vi "Autonomous Independent.vi"() -> ()   [LabVIEW 2012]
doc: "This VI is called when autonomous begins, and will automatically be terminated when autonomous ends. You can carry out timed or sensor driven robot movement independently without needing to return to the caller."
uses:
  <vilib>/Rock Robotics/WPI/Relay/WPI_RelayValue.ctl
  <vilib>/Rock Robotics/WPI/RobotDrive/WPI_RobotDriveGetSetRefNum.vi
  Robot Global Data.vi
panel:
  out "Shooter Up":bool
  out "Shooter Speed":T1(ring)
  out "Stop Drive":bool
  out "DT Output":enum16{"Off", "Up", "Down"}(ring)=enum."Down"
  out "DAD Up":bool
  out "DAD Output":T2
  out "Shift Low":bool
  out "Feeder Happy":bool
  out "Auton Done":bool
  out "Shooter Happy":bool
  out "Shoot!":bool
  out "Delay Switch":u32
  out "Seccond Switch":u32
  out "First Switch":u32
  # "Be sure to right-click and choose Data Operations>>Make Current Value default if you want to save the array values with the VI"
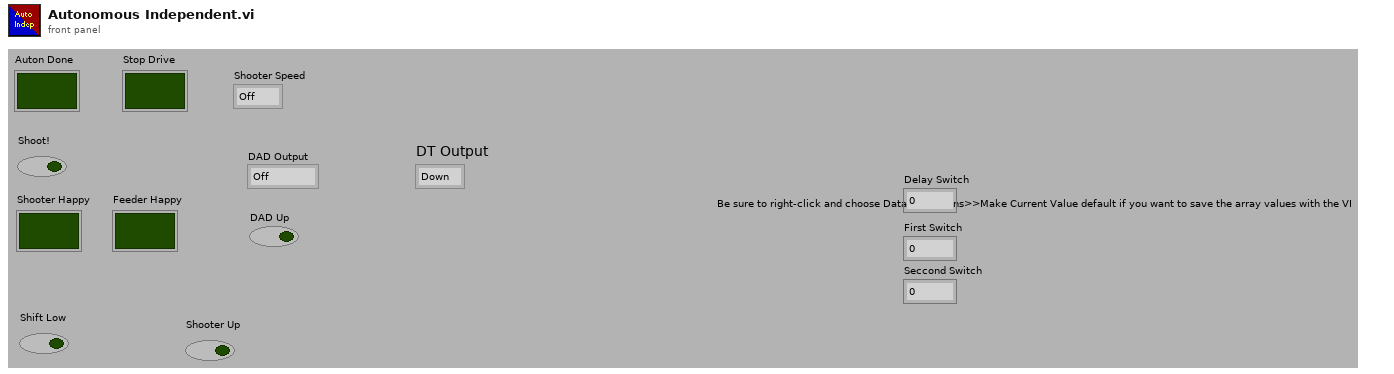
[diagram p1: front panel]
types:
  T1 = enum16{"Off", "Close Pyramid 3pt", "Far Pyramid 3pt", "Feeder Shot", "UD Far 3pt Shot"}
  T2 = typedef "WPI_RelayValue.ctl" = enum16{"Off", "On", "Forward", "Reverse"}
  T3 = enum16{"Off", "Close Pyramid 3pt", "Far Pyramid 3pt", "Feeder Shot"}
  T4 = typedef "WPI_RobotDriveDevRef.ctl" = cluster{"DevStatus":errorcluster, "Motors[]":T5[], "Square Inputs":bool, "Max Output":dbl, "Isochronous":bool}
  T5 = typedef "WPI_MotorControlDeviceRef.ctl" = cluster{"DeviceStatus":errorcluster, "Type":enum16{"PWM", "CAN"}, "PWM":cluster{"Digital Module":T6, "PWM Channel":T7, "DeadBand":T8}, "CAN":cluster{"Device Number":u8, "Control Mode":T9, "Semaphore":T10, "Max Vout":dbl}, "Invert":bool, "TransformRef":T11, "InvTransformRef":T11}
  T6 = typedef "FPGA_TypedefDigitalModule.ctl" = enum16{"Digital Module 1", "Digital Module 2"}
  T7 = typedef "FPGA_DIOPWMChannel.ctl" = enum8{"PWM 1", "PWM 2", "PWM 3", "PWM 4", "PWM 5", "PWM 6", "PWM 7", "PWM 8", "PWM 9", "PWM 10", "Invalid"}
  T8 = typedef "WPI_PWMDeadband.ctl" = cluster{"Name":string, "maxPositivePwm":i32, "minPositivePwm":i32, "centerPwm":i32, "maxNegativePwm":i32, "minNegativePwm":i32, "angularRange":u16}
  T9 = typedef "WPI_CANJaguar_ControlMode.ctl" = enum8{"Percent VBus", "Current", "Speed", "Position", "Voltage"}
  T10 = typedef "Semaphore RefNum" = refnum<k1>
  T11 = typedef "WPI_PWMTransform_ConPane.ctl" = refnum<vi>
  T12 = typedef "WPI_GyroDevRef.ctl" = cluster{"DevStatus":errorcluster, "Analog Module":T13, "Analog Channel":T14, "Offset":dbl, "Gain (VoltsPerDegree/Second)":dbl}
  T13 = typedef "FPGA_TypedefAnalogModule.ctl" = enum16{"Analog Module 1", "Analog Module 2"}
  T14 = typedef "FPGA_AIChannel.ctl" = enum8{"AI 1", "AI 2", "AI 3", "AI 4", "AI 5", "AI 6", "AI 7", "AI 8", "Invalid"}
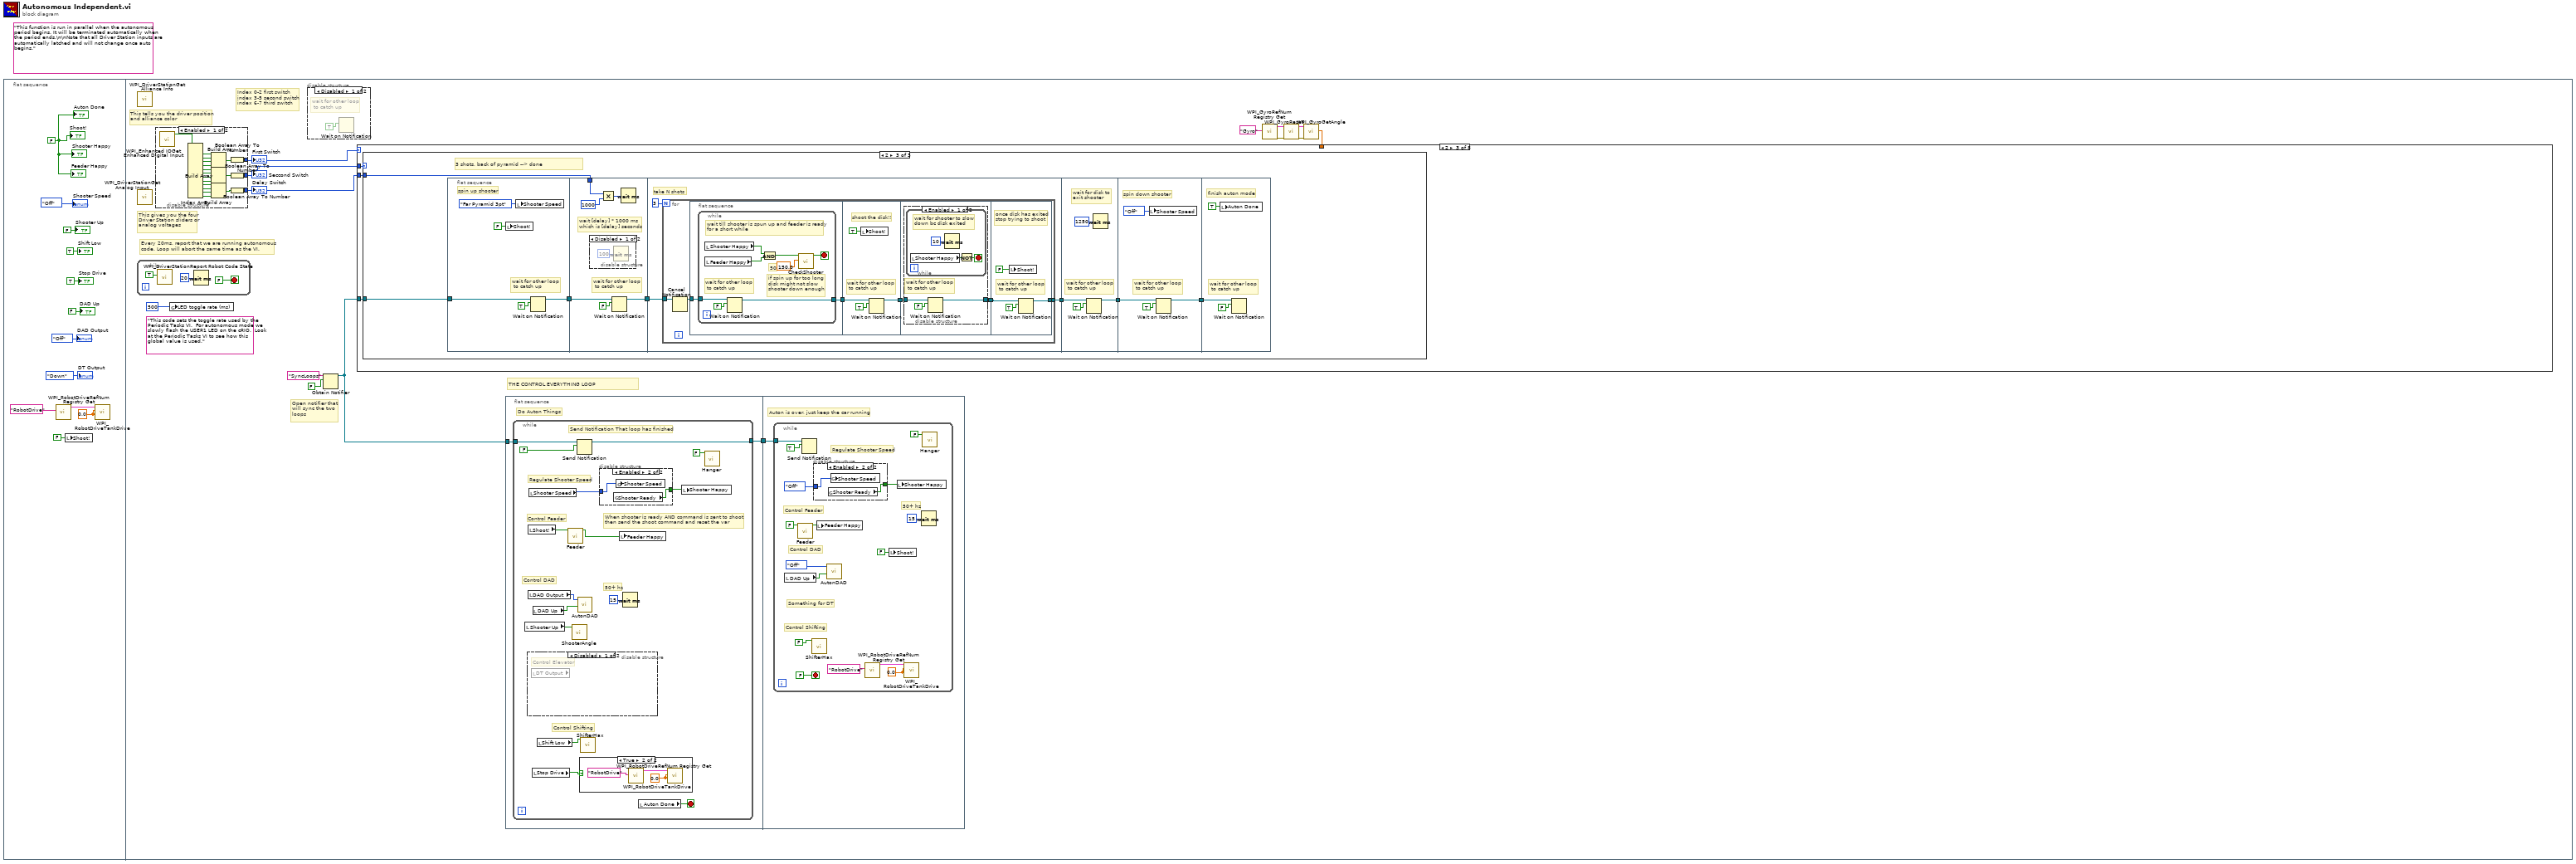
[diagram p0: block diagram]
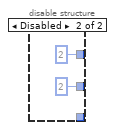
[diagram p2: hidden frame]
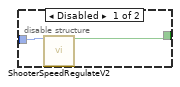
[diagram p4: hidden frame]
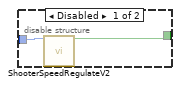
[diagram p7: hidden frame]
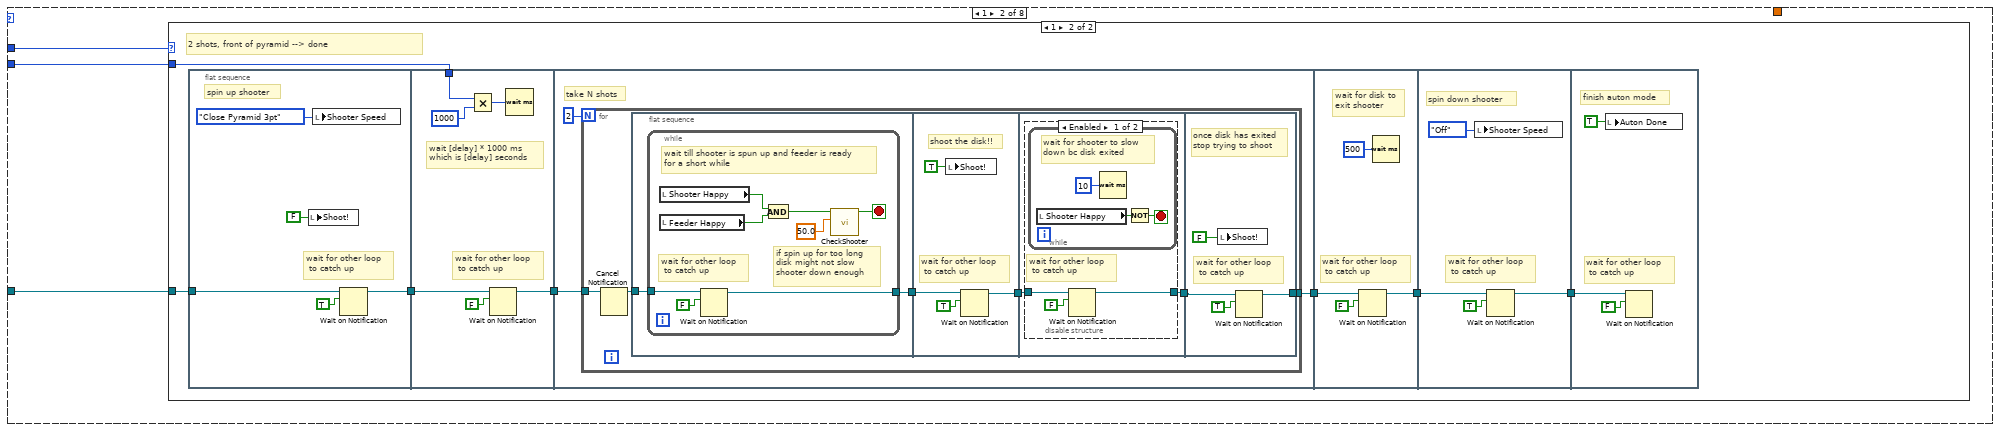
[diagram p9: hidden frame]
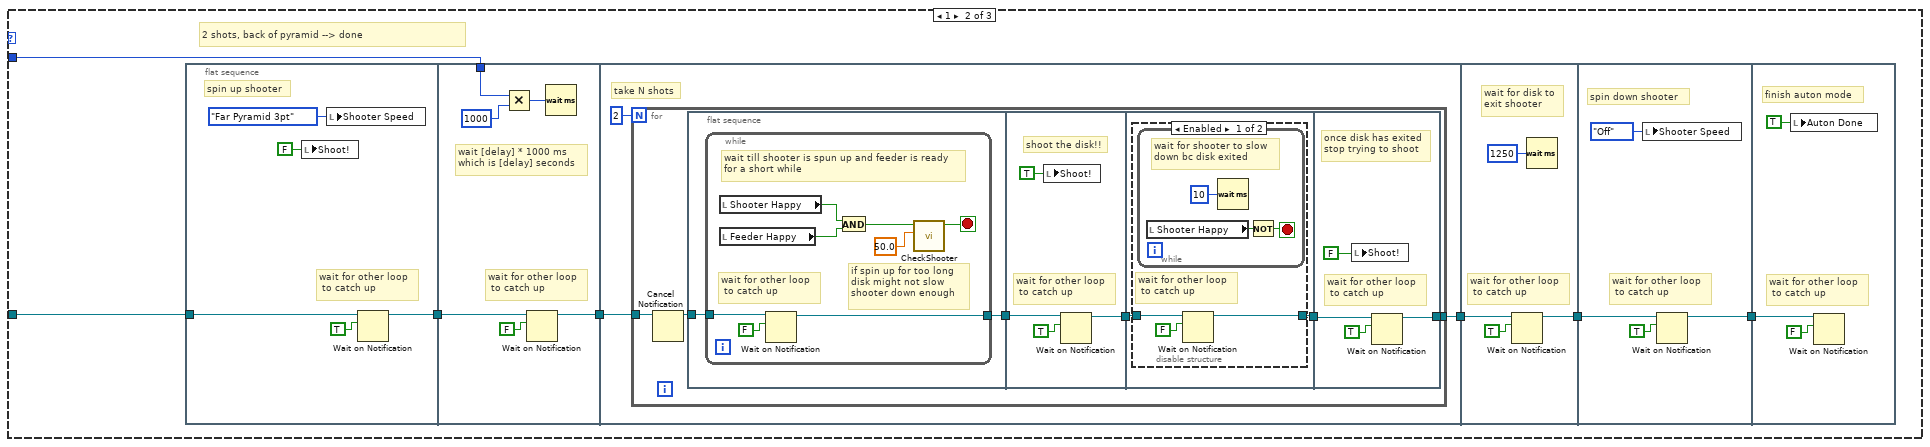
[diagram p13: hidden frame]
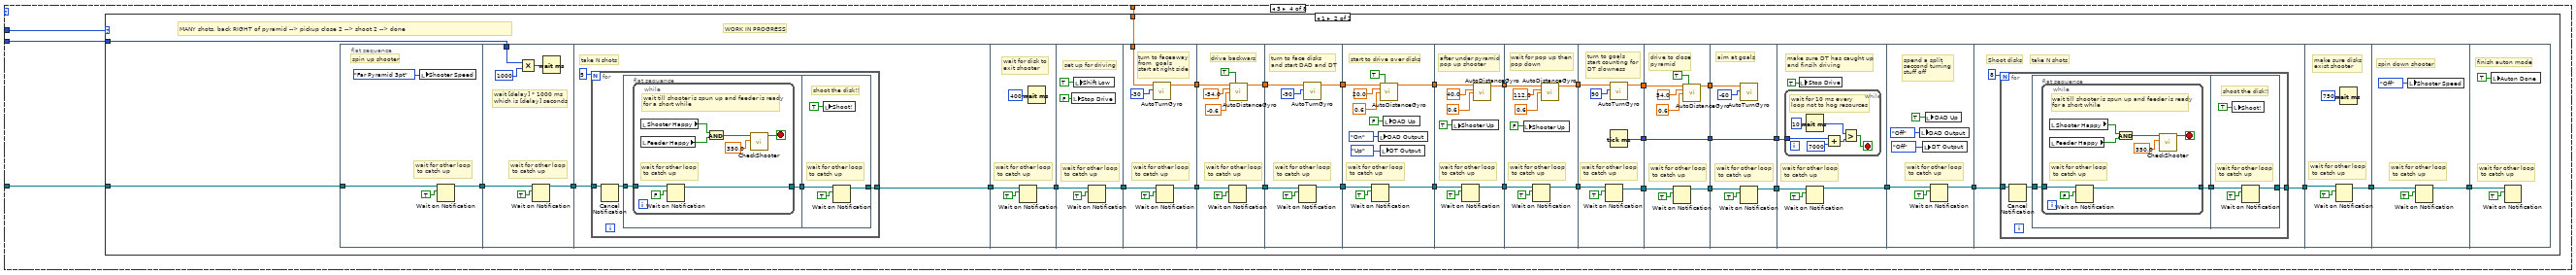
[diagram p17: hidden frame]
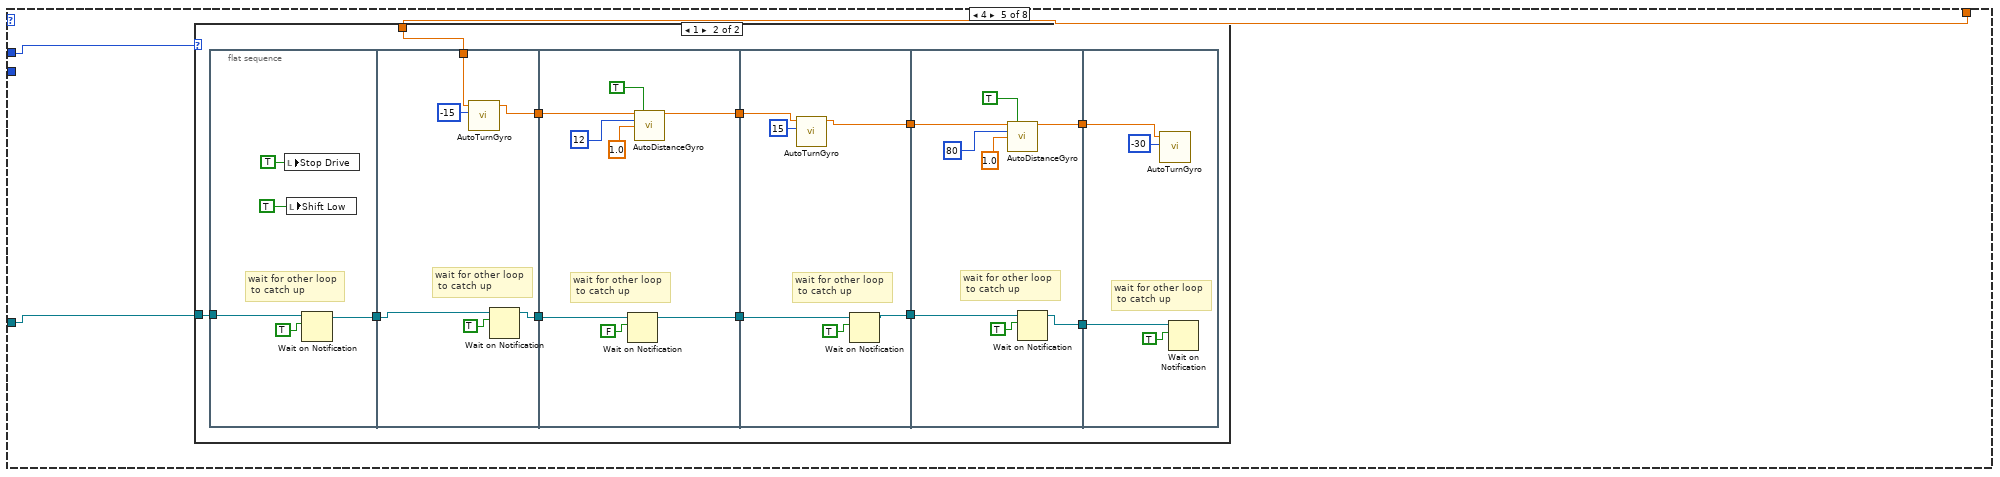
[diagram p19: hidden frame]
diagram:
  (unwired) "This function is run in parallel when the autonomous period begins. It will be terminated automatically when the period ends.\n\nNote that all Driver Station inputs are automatically latched and will not change once auto begins."
  n1 = flat-sequence {
    frame #0 {
      w6 = 0.0 ("Left axis value")
      w12 = FALSE
      n2 = call <vilib>:"WPI_RobotDriveRefNum Registry Get.vi"("refnum name"="RobotDrive") -> ("RobotDriveDevRef"=w7:T4)  [unwired: 1 in, 9 out]
      n3 = local write "Shoot!"(FALSE ("Shoot!")) -> ()
      n4 = call <vilib>:"WPI_RobotDriveTankDrive.vi"("Right axis value"=w6, "Left axis value"=w6, "RobotDriveDevRef"=w7) -> ()  [unwired: 6 in, 3 out]
      "Feeder Happy" <- w12
      "Shift Low" <- TRUE ("Shift Low")
      "DAD Output" <- WPI_RelayValue."Off" ("DAD Output")
      "DAD Up" <- FALSE ("BAD Up")
      "Stop Drive" <- TRUE ("Stop Drive")
      "Shoot!" <- w12
      "Shooter Happy" <- w12
      "Auton Done" <- w12
      "DT Output" <- enum16{"Off", "Up", "Down"}."Down" ("DT Output")
      "Shooter Speed" <- T3."Off" ("Shooter Speed")
      "Shooter Up" <- FALSE ("Shooter Angle")
    }
    frame #1 {
      (unwired) "This code sets the toggle rate used by the Periodic Tasks VI.  For autonomous mode we slowly flash the USER1 LED on the cRIO.  Look at the Periodic Tasks VI to see how this global value is used."
      # "THE CONTROL EVERYTHING LOOP"
      # "Index 0-2 first switch\nindex 3-5 second switch\nindex 6-7 third switch"
      # "Open notifier that\nwill sync the two\nloops"
      # "Every 20ms, report that we are running autonomous\ncode. Loop will abort the same time as the VI."
      # "This tells you the driver position\nand alliance color"
      # "This gives you the four\nDriver Station sliders or\nanalog voltages"
      n5 = call <vilib>:"WPI_DriverStationGet Alliance Info.vi"() -> ()  [unwired: 12 out]
      n6 = call <vilib>:"WPI_DriverStationGet Analog Input.vi"() -> ()  [unwired: 12 out]
      n7 = while {
        stop <- FALSE stop-if-true
        n8 = call <vilib>:"WPI_DriverStationReport Robot Code State.vi"("Autonomous"=TRUE) -> ()  [unwired: 10 in, 1 out]
        n9 = Wait (ms)(milliseconds to wait=u32 20) -> ()  [unwired: 1 out]
      }
      n10 = disable-structure shown="Enabled" {
        disable-tunnel: [w29 u32 2 ("First Switch")] -> w21
        disable-tunnel: [w28 u32 2 ("Seccond Switch")] -> w20
        disable-tunnel: [w27 _] -> w18
        frame Enabled {
          n11 = call <vilib>:"WPI_Enhanced IOGet Enhanced Digital Input.vi"() -> ("Digital Input [1-16]"=w30:bool[])  [unwired: 10 in, 1 out]
          n12 = Index Array(array=w30) -> (element #1=w45:bool, element #2=w44:bool, element #3=w43:bool, element #4=w36:bool, element #5=w42:bool, element #6=w41:bool, element #7=w38:bool, element #8=w37:bool, element #9=w35:bool, element #10=w34:bool, element #11=w33:bool, element #12=w32:bool)  [unwired: 12 in]
          n13 = Build Array(w45, w44, w43, w36) -> (w39:bool[])
          n14 = Build Array(w42, w41, w38, w37) -> (w40:bool[])
          n15 = Build Array(w35, w34, w33, w32) -> (w31:bool[])
          n16 = Boolean Array To Number(Boolean array=w39) -> (number=w29:u32)
          n17 = Boolean Array To Number(Boolean array=w40) -> (number=w28:u32)
          n18 = Boolean Array To Number(Boolean array=w31) -> (number=w27:u32)
        }
        frame Disabled {
        }
      }
      "First Switch" <- w21
      "Seccond Switch" <- w20
      "Delay Switch" <- w18
      n19 = global write "Robot Global Data.vi" "LED toggle rate (ms)"(u32 500 ("LED ms toggle rate")) -> ()
      n20 = disable-structure shown="Disabled" {
        frame Disabled {
          # "wait for other loop\n to catch up"
          n21 = Wait on Notification(ignore previous (F)=TRUE) -> (notifier=w49:refnum<notifier>)  [unwired: 2 in, 4 out]
        }
        frame Enabled {
        }
      }
      n22 = Obtain Notifier(name (unnamed)="SyncLoops", notification data type=FALSE) -> (notifier out=w19:refnum<notifier>)  [unwired: 2 in, 2 out]
      n23 = flat-sequence {
        tunnel: w19 -> [w51]
        tunnel: [w50] -> w26
        tunnel: w26 -> [w74]
        frame #0 {
          # "Do Auton Things"
          n24 = while {
            tunnel: w51 -> [w64]
            tunnel: [w62] -> w50
            stop <- w66 stop-if-true
            # "Regulate Shooter Speed"
            # "50+ hz"
            # "Control DAD"
            # "Control Shifting"
            # "When shooter is ready AND command is sent to shoot\nthen send the shoot command and reset the var"
            # "Control Feader"
            # "Send Notification That loop has finished"
            n25 = local read "Shooter Up"() -> (w53:bool)
            n26 = disable-structure shown="Disabled" {
              frame Disabled {
                # "Control Elevator"
                n27 = local read "DT Output"() -> ()  [unwired: 1 out]
              }
              frame Enabled {
              }
            }
            n28 = local read "Shoot!"() -> (w52:bool)
            n29 = local read "DAD Output"() -> (w58:T2)
            n30 = local read "Shooter Speed"() -> (w55:T1)
            n31 = local read "Stop Drive"() -> (w60:bool)
            n32 = local read "DAD Up"() -> (w59:bool)
            n33 = local read "Shift Low"() -> (w56:bool)
            n34 = call "Feeder.vi"("SHOOT Button"=w52) -> ("Ready To Shoot?"=w63:bool)  [unwired: 10 in]
            n35 = call "ShooterAngle.vi"("Shooter Angle Up?"=w53) -> ()  [unwired: 10 in, 1 out]
            n36 = Send Notification(notification=FALSE, notifier=w64) -> (notifier out=w62:refnum<notifier>)  [unwired: 1 in, 1 out]
            n37 = call "AutonDAD.vi"("BAD UP"=w59, "BAD Output"=w58) -> ()  [unwired: 10 in]
            n38 = case shown="True" w60 {
              frame False {
              }
              frame True {
                w73 = 0.0 ("Left axis value")
                n39 = call <vilib>:"WPI_RobotDriveRefNum Registry Get.vi"("refnum name"="RobotDrive") -> ("RobotDriveDevRef"=w72:T4)  [unwired: 1 in, 9 out]
                n40 = call <vilib>:"WPI_RobotDriveTankDrive.vi"("Right axis value"=w73, "Left axis value"=w73, "RobotDriveDevRef"=w72) -> ()  [unwired: 6 in, 3 out]
              }
            }
            n41 = call "ShifterHax.vi"("Shift low?"=w56) -> ()  [unwired: 11 in]
            n42 = disable-structure shown="Enabled" {
              disable-tunnel: [w68 w69] -> w57
              disable-tunnel: w55 -> [w67 w70]
              frame Disabled {
                n43 = call "ShooterSpeedRegulateV2.vi"("Shooter Speed"=w67) -> ("ALL GOOD"=w68:bool)  [unwired: 13 in, 1 out]
              }
              frame Enabled {
                n44 = global read "Robot Global Data.vi" "Shooter Ready"() -> (w69:bool)
                n45 = global write "Robot Global Data.vi" "Shooter Speed"(w70) -> ()
              }
            }
            n46 = local write "Feeder Happy"(w63) -> ()
            n47 = Wait (ms)(milliseconds to wait=u32 15) -> ()  [unwired: 1 out]
            n48 = local read "Auton Done"() -> (w66:bool)
            n49 = local write "Shooter Happy"(w57) -> ()
            n50 = call "Hanger.vi"("Hanger Up"=FALSE) -> ()  [unwired: 10 in, 1 out]
          }
        }
        frame #1 {
          # "Auton is over, just keep the car running"
          n51 = while {
            tunnel: w74 -> [w81]
            stop <- FALSE stop-if-true
            w86 = 0.0 ("Left axis value")
            # "Something for DT"
            # "50+ hz"
            # "Regulate Shooter Speed"
            # "Control DAD"
            # "Control Shifting"
            # "Control Feader"
            n52 = local read "DAD Up"() -> (w84:bool)
            n53 = call "Feeder.vi"("SHOOT Button"=FALSE) -> ("Ready To Shoot?"=w89:bool)  [unwired: 10 in]
            n54 = Send Notification(notification=TRUE, notifier=w81) -> ()  [unwired: 1 in, 2 out]
            n55 = call "ShifterHax.vi"("Shift low?"=FALSE ("Shifting Button")) -> ()  [unwired: 11 in]
            n56 = disable-structure shown="Enabled" {
              disable-tunnel: [w92 w93] -> w78
              disable-tunnel: T3."Off" ("Shooter Speed") -> [w91 w94]
              frame Disabled {
                n57 = call "ShooterSpeedRegulateV2.vi"("Shooter Speed"=w91) -> ("ALL GOOD"=w92:bool)  [unwired: 13 in, 1 out]
              }
              frame Enabled {
                n58 = global read "Robot Global Data.vi" "Shooter Ready"() -> (w93:bool)
                n59 = global write "Robot Global Data.vi" "Shooter Speed"(w94) -> ()
              }
            }
            n60 = local write "Feeder Happy"(w89) -> ()
            n61 = call "AutonDAD.vi"("BAD UP"=w84, "BAD Output"=WPI_RelayValue."Off") -> ()  [unwired: 10 in]
            n62 = call <vilib>:"WPI_RobotDriveRefNum Registry Get.vi"("refnum name"="RobotDrive") -> ("RobotDriveDevRef"=w87:T4)  [unwired: 1 in, 9 out]
            n63 = local write "Shoot!"(FALSE ("Shoot!")) -> ()
            n64 = local write "Shooter Happy"(w78) -> ()
            n65 = call <vilib>:"WPI_RobotDriveTankDrive.vi"("Right axis value"=w86, "Left axis value"=w86, "RobotDriveDevRef"=w87) -> ()  [unwired: 6 in, 3 out]
            n66 = Wait (ms)(milliseconds to wait=u32 15) -> ()  [unwired: 1 out]
            n67 = call "Hanger.vi"("Hanger Up"=FALSE) -> ()  [unwired: 10 in, 1 out]
          }
        }
      }
      n68 = call <vilib>:"WPI_GyroRefNum Registry Get.vi"("refnum name"="Gyro") -> ("error out"=w17:errorcluster, "GyroDevRef"=w16:T12)  [unwired: 9 in]
      n69 = call <vilib>:"WPI_GyroReset.vi"("error in (no error)"=w17, "GyroDevRef"=w16) -> ("error out"=w15:errorcluster, "GyroDevRef"=w14:T12)  [unwired: 8 in]
      n70 = call <vilib>:"WPI_GyroGetAngle.vi"("error in (no error)"=w15, "GyroDevRef"=w14) -> ("Angle"=w13:dbl)  [unwired: 6 in, 3 out]
      n71 = case shown="2" w21 {
        tunnel: w20 -> [_ w97 w164 w297 w491 w543 w722 w902]
        tunnel: w19 -> [_ w96 w163 w296 w490 w542 w721 w901]
        tunnel: w18 -> [_ w95 w162 w295 _ w541 w720 _]
        tunnel: w13 -> [_ _ _ w294 w489 w540 w719 w900]
        frame 0, Default {
          # "do nothing"
        }
        frame 1 {
          n72 = case shown="1" w97 {
            tunnel: w96 -> [_ w101]
            tunnel: w95 -> [_ w104]
            frame 0, Default {
              # "do nothing"
            }
            frame 1 {
              # "2 shots, front of pyramid --> done"
              n73 = flat-sequence {
                tunnel: [w108] -> w103
                tunnel: w101 -> [w107]
                tunnel: w104 -> [w113]
                tunnel: w103 -> [w111]
                tunnel: [w110] -> w102
                tunnel: w102 -> [w117]
                tunnel: [w116] -> w98
                tunnel: [w152] -> w99
                tunnel: w98 -> [w151]
                tunnel: [w157] -> w100
                tunnel: w99 -> [w156]
                tunnel: w100 -> [w159]
                frame #0 {
                  # "wait for other loop\n to catch up"
                  # "spin up shooter"
                  n74 = local write "Shoot!"(FALSE ("Shoot!")) -> ()
                  n75 = local write "Shooter Speed"(T3."Close Pyramid 3pt" ("Shooter Speed")) -> ()
                  n76 = Wait on Notification(notifier=w107, ignore previous (F)=TRUE) -> (notifier out=w108:refnum<notifier>)  [unwired: 2 in, 3 out]
                }
                frame #1 {
                  # "wait for other loop\n to catch up"
                  # "wait [delay] * 1000 ms\nwhich is [delay] seconds"
                  n77 = Multiply(x=w113, y=1000) -> (x*y=w115:u32)
                  n78 = Wait on Notification(notifier=w111, ignore previous (F)=FALSE) -> (notifier out=w110:refnum<notifier>)  [unwired: 2 in, 3 out]
                  n79 = Wait (ms)(milliseconds to wait=w115) -> ()  [unwired: 1 out]
                }
                frame #2 {
                  # "take N shots"
                  n80 = for {
                    N: 2 -> [_]
                    tunnel: w117 -> [w123]
                    tunnel: [w121] -> w116
                    n81 = Cancel Notification(0:w123) -> (8:w124:refnum<notifier>)  [unwired: 1 in, 2 out]
                    n82 = flat-sequence {
                      tunnel: w124 -> [w126]
                      tunnel: [w125] -> w122
                      tunnel: w122 -> [w136]
                      tunnel: [w135] -> w120
                      tunnel: w120 -> [w139]
                      tunnel: [w140] -> w119
                      tunnel: [w149] -> w121
                      tunnel: w119 -> [w148]
                      frame #0 {
                        n83 = while {
                          tunnel: w126 -> [w128]
                          tunnel: [w127] -> w125
                          stop <- w130 stop-if-true
                          # "if spin up for too long\ndisk might not slow\nshooter down enough"
                          # "wait for other loop\n to catch up"
                          # "wait till shooter is spun up and feeder is ready\nfor a short while"
                          n84 = local read "Shooter Happy"() -> (w133:bool)
                          n85 = local read "Feeder Happy"() -> (w132:bool)
                          n86 = Wait on Notification(notifier=w128, ignore previous (F)=FALSE) -> (notifier out=w127:refnum<notifier>)  [unwired: 2 in, 3 out]
                          n87 = And(x=w133, y=w132) -> (x .and. y?=w131:bool)
                          n88 = call "CheckShooter.vi"("Time for happy (ms)"=50.0, "Shooter Good?"=w131) -> ("Good to shoot"=w130:bool)  [unwired: 9 in]
                        }
                      }
                      frame #1 {
                        # "wait for other loop\n to catch up"
                        # "shoot the disk!!"
                        n89 = local write "Shoot!"(TRUE ("Shoot!")) -> ()
                        n90 = Wait on Notification(notifier=w136, ignore previous (F)=TRUE) -> (notifier out=w135:refnum<notifier>)  [unwired: 2 in, 3 out]
                      }
                      frame #2 {
                        n91 = disable-structure shown="Enabled" {
                          disable-tunnel: [w142 _] -> w140
                          disable-tunnel: w139 -> [w141 _]
                          frame Enabled {
                            # "wait for other loop\n to catch up"
                            n92 = while {
                              stop <- w146 stop-if-true
                              # "wait for shooter to slow\ndown bc disk exited"
                              n93 = local read "Shooter Happy"() -> (w145:bool)
                              n94 = Wait (ms)(milliseconds to wait=u32 10) -> ()  [unwired: 1 out]
                              n95 = Not(x=w145) -> (.not. x?=w146:bool)
                            }
                            n96 = Wait on Notification(notifier=w141, ignore previous (F)=FALSE) -> (notifier out=w142:refnum<notifier>)  [unwired: 2 in, 3 out]
                          }
                          frame Disabled {
                          }
                        }
                      }
                      frame #3 {
                        # "once disk has exited\nstop trying to shoot"
                        # "wait for other loop\n to catch up"
                        n97 = local write "Shoot!"(FALSE) -> ()
                        n98 = Wait on Notification(notifier=w148, ignore previous (F)=TRUE) -> (notifier out=w149:refnum<notifier>)  [unwired: 2 in, 3 out]
                      }
                    }
                  }
                }
                frame #3 {
                  # "wait for other loop\n to catch up"
                  # "wait for disk to\nexit shooter"
                  n99 = Wait on Notification(notifier=w151, ignore previous (F)=FALSE) -> (notifier out=w152:refnum<notifier>)  [unwired: 2 in, 3 out]
                  n100 = Wait (ms)(milliseconds to wait=u32 500) -> ()  [unwired: 1 out]
                }
                frame #4 {
                  # "wait for other loop\n to catch up"
                  # "spin down shooter"
                  n101 = local write "Shooter Speed"(T3."Off" ("Shooter Speed")) -> ()
                  n102 = Wait on Notification(notifier=w156, ignore previous (F)=TRUE) -> (notifier out=w157:refnum<notifier>)  [unwired: 2 in, 3 out]
                }
                frame #5 {
                  # "wait for other loop\n to catch up"
                  # "finish auton mode"
                  n103 = local write "Auton Done"(TRUE ("Auton Done")) -> ()
                  n104 = Wait on Notification(notifier=w159, ignore previous (F)=FALSE) -> ()  [unwired: 2 in, 4 out]
                }
              }
            }
          }
        }
        frame 2 {
          n105 = case shown="2" w164 {
            tunnel: w163 -> [_ w168 w232]
            tunnel: w162 -> [_ w171 w235]
            frame 0, Default {
              # "do nothing"
            }
            frame 1 {
              # "2 shots, back of pyramid --> done"
              n106 = flat-sequence {
                tunnel: [w175] -> w170
                tunnel: w168 -> [w174]
                tunnel: w171 -> [w180]
                tunnel: w170 -> [w178]
                tunnel: [w177] -> w169
                tunnel: w169 -> [w184]
                tunnel: [w183] -> w165
                tunnel: [w219] -> w166
                tunnel: w165 -> [w218]
                tunnel: [w224] -> w167
                tunnel: w166 -> [w223]
                tunnel: w167 -> [w226]
                frame #0 {
                  # "wait for other loop\n to catch up"
                  # "spin up shooter"
                  n107 = local write "Shoot!"(FALSE ("Shoot!")) -> ()
                  n108 = local write "Shooter Speed"(T1."Far Pyramid 3pt" ("Shooter Speed")) -> ()
                  n109 = Wait on Notification(notifier=w174, ignore previous (F)=TRUE) -> (notifier out=w175:refnum<notifier>)  [unwired: 2 in, 3 out]
                }
                frame #1 {
                  # "wait for other loop\n to catch up"
                  # "wait [delay] * 1000 ms\nwhich is [delay] seconds"
                  n110 = Multiply(x=w180, y=1000) -> (x*y=w182:u32)
                  n111 = Wait on Notification(notifier=w178, ignore previous (F)=FALSE) -> (notifier out=w177:refnum<notifier>)  [unwired: 2 in, 3 out]
                  n112 = Wait (ms)(milliseconds to wait=w182) -> ()  [unwired: 1 out]
                }
                frame #2 {
                  # "take N shots"
                  n113 = for {
                    N: 2 -> [_]
                    tunnel: w184 -> [w190]
                    tunnel: [w188] -> w183
                    n114 = Cancel Notification(0:w190) -> (8:w191:refnum<notifier>)  [unwired: 1 in, 2 out]
                    n115 = flat-sequence {
                      tunnel: w191 -> [w193]
                      tunnel: [w192] -> w189
                      tunnel: w189 -> [w203]
                      tunnel: [w202] -> w187
                      tunnel: w187 -> [w206]
                      tunnel: [w207] -> w186
                      tunnel: [w216] -> w188
                      tunnel: w186 -> [w215]
                      frame #0 {
                        n116 = while {
                          tunnel: w193 -> [w195]
                          tunnel: [w194] -> w192
                          stop <- w197 stop-if-true
                          # "if spin up for too long\ndisk might not slow\nshooter down enough"
                          # "wait for other loop\n to catch up"
                          # "wait till shooter is spun up and feeder is ready\nfor a short while"
                          n117 = local read "Shooter Happy"() -> (w200:bool)
                          n118 = local read "Feeder Happy"() -> (w199:bool)
                          n119 = Wait on Notification(notifier=w195, ignore previous (F)=FALSE) -> (notifier out=w194:refnum<notifier>)  [unwired: 2 in, 3 out]
                          n120 = And(x=w200, y=w199) -> (x .and. y?=w198:bool)
                          n121 = call "CheckShooter.vi"("Time for happy (ms)"=50.0, "Shooter Good?"=w198) -> ("Good to shoot"=w197:bool)  [unwired: 9 in]
                        }
                      }
                      frame #1 {
                        # "wait for other loop\n to catch up"
                        # "shoot the disk!!"
                        n122 = local write "Shoot!"(TRUE ("Shoot!")) -> ()
                        n123 = Wait on Notification(notifier=w203, ignore previous (F)=TRUE) -> (notifier out=w202:refnum<notifier>)  [unwired: 2 in, 3 out]
                      }
                      frame #2 {
                        n124 = disable-structure shown="Enabled" {
                          disable-tunnel: [w209 _] -> w207
                          disable-tunnel: w206 -> [w208 _]
                          frame Enabled {
                            # "wait for other loop\n to catch up"
                            n125 = while {
                              stop <- w213 stop-if-true
                              # "wait for shooter to slow\ndown bc disk exited"
                              n126 = local read "Shooter Happy"() -> (w212:bool)
                              n127 = Wait (ms)(milliseconds to wait=u32 10) -> ()  [unwired: 1 out]
                              n128 = Not(x=w212) -> (.not. x?=w213:bool)
                            }
                            n129 = Wait on Notification(notifier=w208, ignore previous (F)=FALSE) -> (notifier out=w209:refnum<notifier>)  [unwired: 2 in, 3 out]
                          }
                          frame Disabled {
                          }
                        }
                      }
                      frame #3 {
                        # "once disk has exited\nstop trying to shoot"
                        # "wait for other loop\n to catch up"
                        n130 = local write "Shoot!"(FALSE) -> ()
                        n131 = Wait on Notification(notifier=w215, ignore previous (F)=TRUE) -> (notifier out=w216:refnum<notifier>)  [unwired: 2 in, 3 out]
                      }
                    }
                  }
                }
                frame #3 {
                  # "wait for other loop\n to catch up"
                  # "wait for disk to\nexit shooter"
                  n132 = Wait on Notification(notifier=w218, ignore previous (F)=TRUE) -> (notifier out=w219:refnum<notifier>)  [unwired: 2 in, 3 out]
                  n133 = Wait (ms)(milliseconds to wait=u32 1250) -> ()  [unwired: 1 out]
                }
                frame #4 {
                  # "wait for other loop\n to catch up"
                  # "spin down shooter"
                  n134 = local write "Shooter Speed"(T3."Off" ("Shooter Speed")) -> ()
                  n135 = Wait on Notification(notifier=w223, ignore previous (F)=TRUE) -> (notifier out=w224:refnum<notifier>)  [unwired: 2 in, 3 out]
                }
                frame #5 {
                  # "wait for other loop\n to catch up"
                  # "finish auton mode"
                  n136 = local write "Auton Done"(TRUE ("Auton Done")) -> ()
                  n137 = Wait on Notification(notifier=w226, ignore previous (F)=FALSE) -> ()  [unwired: 2 in, 4 out]
                }
              }
            }
            frame 2 {
              # "3 shots, back of pyramid --> done"
              n138 = flat-sequence {
                tunnel: [w239] -> w234
                tunnel: w232 -> [w238]
                tunnel: w235 -> [w244]
                tunnel: w234 -> [w242]
                tunnel: [w241] -> w233
                tunnel: w233 -> [w249]
                tunnel: [w248] -> w229
                tunnel: [w284] -> w230
                tunnel: w229 -> [w283]
                tunnel: [w289] -> w231
                tunnel: w230 -> [w288]
                tunnel: w231 -> [w291]
                frame #0 {
                  # "wait for other loop\n to catch up"
                  # "spin up shooter"
                  n139 = local write "Shoot!"(FALSE ("Shoot!")) -> ()
                  n140 = local write "Shooter Speed"(T1."Far Pyramid 3pt" ("Shooter Speed")) -> ()
                  n141 = Wait on Notification(notifier=w238, ignore previous (F)=TRUE) -> (notifier out=w239:refnum<notifier>)  [unwired: 2 in, 3 out]
                }
                frame #1 {
                  # "wait for other loop\n to catch up"
                  # "wait [delay] * 1000 ms\nwhich is [delay] seconds"
                  n142 = disable-structure shown="Disabled" {
                    frame Disabled {
                      n143 = Wait (ms)(milliseconds to wait=u32 100) -> ()  [unwired: 1 out]
                    }
                    frame Enabled {
                    }
                  }
                  n144 = Multiply(x=w244, y=1000) -> (x*y=w246:u32)
                  n145 = Wait on Notification(notifier=w242, ignore previous (F)=FALSE) -> (notifier out=w241:refnum<notifier>)  [unwired: 2 in, 3 out]
                  n146 = Wait (ms)(milliseconds to wait=w246) -> ()  [unwired: 1 out]
                }
                frame #2 {
                  # "take N shots"
                  n147 = for {
                    N: 3 -> [_]
                    tunnel: w249 -> [w255]
                    tunnel: [w253] -> w248
                    n148 = Cancel Notification(0:w255) -> (8:w256:refnum<notifier>)  [unwired: 1 in, 2 out]
                    n149 = flat-sequence {
                      tunnel: w256 -> [w258]
                      tunnel: [w257] -> w254
                      tunnel: w254 -> [w268]
                      tunnel: [w267] -> w252
                      tunnel: w252 -> [w271]
                      tunnel: [w272] -> w251
                      tunnel: [w281] -> w253
                      tunnel: w251 -> [w280]
                      frame #0 {
                        n150 = while {
                          tunnel: w258 -> [w260]
                          tunnel: [w259] -> w257
                          stop <- w262 stop-if-true
                          # "50"
                          # "if spin up for too long\ndisk might not slow\nshooter down enough"
                          # "wait for other loop\n to catch up"
                          # "wait till shooter is spun up and feeder is ready\nfor a short while"
                          n151 = local read "Shooter Happy"() -> (w265:bool)
                          n152 = local read "Feeder Happy"() -> (w264:bool)
                          n153 = Wait on Notification(notifier=w260, ignore previous (F)=FALSE) -> (notifier out=w259:refnum<notifier>)  [unwired: 2 in, 3 out]
                          n154 = And(x=w265, y=w264) -> (x .and. y?=w263:bool)
                          n155 = call "CheckShooter.vi"("Time for happy (ms)"=150.0, "Shooter Good?"=w263) -> ("Good to shoot"=w262:bool)  [unwired: 9 in]
                        }
                      }
                      frame #1 {
                        # "wait for other loop\n to catch up"
                        # "shoot the disk!!"
                        n156 = local write "Shoot!"(TRUE ("Shoot!")) -> ()
                        n157 = Wait on Notification(notifier=w268, ignore previous (F)=TRUE) -> (notifier out=w267:refnum<notifier>)  [unwired: 2 in, 3 out]
                      }
                      frame #2 {
                        n158 = disable-structure shown="Enabled" {
                          disable-tunnel: [w274 _] -> w272
                          disable-tunnel: w271 -> [w273 _]
                          frame Enabled {
                            # "wait for other loop\n to catch up"
                            n159 = while {
                              stop <- w278 stop-if-true
                              # "wait for shooter to slow\ndown bc disk exited"
                              n160 = local read "Shooter Happy"() -> (w277:bool)
                              n161 = Wait (ms)(milliseconds to wait=u32 10) -> ()  [unwired: 1 out]
                              n162 = Not(x=w277) -> (.not. x?=w278:bool)
                            }
                            n163 = Wait on Notification(notifier=w273, ignore previous (F)=FALSE) -> (notifier out=w274:refnum<notifier>)  [unwired: 2 in, 3 out]
                          }
                          frame Disabled {
                          }
                        }
                      }
                      frame #3 {
                        # "once disk has exited\nstop trying to shoot"
                        # "wait for other loop\n to catch up"
                        n164 = local write "Shoot!"(FALSE) -> ()
                        n165 = Wait on Notification(notifier=w280, ignore previous (F)=TRUE) -> (notifier out=w281:refnum<notifier>)  [unwired: 2 in, 3 out]
                      }
                    }
                  }
                }
                frame #3 {
                  # "wait for other loop\n to catch up"
                  # "wait for disk to\nexit shooter"
                  n166 = Wait on Notification(notifier=w283, ignore previous (F)=TRUE) -> (notifier out=w284:refnum<notifier>)  [unwired: 2 in, 3 out]
                  n167 = Wait (ms)(milliseconds to wait=u32 1250) -> ()  [unwired: 1 out]
                }
                frame #4 {
                  # "wait for other loop\n to catch up"
                  # "spin down shooter"
                  n168 = local write "Shooter Speed"(T3."Off" ("Shooter Speed")) -> ()
                  n169 = Wait on Notification(notifier=w288, ignore previous (F)=TRUE) -> (notifier out=w289:refnum<notifier>)  [unwired: 2 in, 3 out]
                }
                frame #5 {
                  # "wait for other loop\n to catch up"
                  # "finish auton mode"
                  n170 = local write "Auton Done"(TRUE ("Auton Done")) -> ()
                  n171 = Wait on Notification(notifier=w291, ignore previous (F)=FALSE) -> ()  [unwired: 2 in, 4 out]
                }
              }
            }
          }
        }
        frame 3 {
          n172 = case shown="1" w297 {
            tunnel: w296 -> [_ w327]
            tunnel: w295 -> [_ w330]
            tunnel: w294 -> [_ w319]
            frame 0, Default {
              # "do nothing"
            }
            frame 1 {
              # "WORK IN PROGRESS"
              # "MANY shots, back RIGHT of pyramid --> pickup close 2 --> shoot 2 --> done"
              n173 = flat-sequence {
                tunnel: [w333] -> w329
                tunnel: w327 -> [w332]
                tunnel: w330 -> [w338]
                tunnel: w329 -> [w336]
                tunnel: [w335] -> w328
                tunnel: w328 -> [w342]
                tunnel: [w341] -> w325
                tunnel: [w363] -> w324
                tunnel: w325 -> [w362]
                tunnel: w324 -> [w366]
                tunnel: [w367] -> w323
                tunnel: [w375] -> w322
                tunnel: w323 -> [w374]
                tunnel: w319 -> [w373]
                tunnel: [w371] -> w318
                tunnel: w322 -> [w382]
                tunnel: [w383] -> w320
                tunnel: w318 -> [w381]
                tunnel: [w380] -> w317
                tunnel: [w389] -> w321
                tunnel: w320 -> [w388]
                tunnel: w317 -> [w386]
                tunnel: [w385] -> w316
                tunnel: [w400] -> w301
                tunnel: w321 -> [w399]
                tunnel: w316 -> [w396]
                tunnel: [w395] -> w299
                tunnel: w301 -> [w408]
                tunnel: [w407] -> w300
                tunnel: w299 -> [w404]
                tunnel: [w403] -> w298
                tunnel: w300 -> [w415]
                tunnel: [w416] -> w303
                tunnel: [w411] -> w302
                tunnel: w298 -> [w412]
                tunnel: [w423] -> w313
                tunnel: w303 -> [w422]
                tunnel: w302 -> [w420]
                tunnel: [w419] -> w312
                tunnel: [w418] -> w311
                tunnel: w313 -> [w430]
                tunnel: [w431] -> w310
                tunnel: w312 -> [w433]
                tunnel: [w433] -> w308
                tunnel: w311 -> [w427]
                tunnel: [w425] -> w306
                tunnel: w310 -> [w436]
                tunnel: [w437] -> w309
                tunnel: w308 -> [w439]
                tunnel: [w439] -> w307
                tunnel: w306 -> [w434]
                tunnel: [w443] -> w305
                tunnel: w309 -> [w442]
                tunnel: w307 -> [w441]
                tunnel: w305 -> [w454]
                tunnel: [w455] -> w304
                tunnel: [w458] -> w315
                tunnel: w304 -> [w457]
                tunnel: w315 -> [w479]
                tunnel: [w480] -> w314
                tunnel: [w484] -> w326
                tunnel: w314 -> [w483]
                tunnel: w326 -> [w486]
                frame #0 {
                  # "wait for other loop\n to catch up"
                  # "spin up shooter"
                  n174 = local write "Shooter Speed"(T3."Far Pyramid 3pt" ("Shooter Speed")) -> ()
                  n175 = Wait on Notification(notifier=w332, ignore previous (F)=TRUE) -> (notifier out=w333:refnum<notifier>)  [unwired: 2 in, 3 out]
                }
                frame #1 {
                  # "wait for other loop\n to catch up"
                  # "wait [delay] * 1000 ms\nwhich is [delay] seconds"
                  n176 = Multiply(x=w338, y=1000) -> (x*y=w340:u32)
                  n177 = Wait on Notification(notifier=w336, ignore previous (F)=TRUE) -> (notifier out=w335:refnum<notifier>)  [unwired: 2 in, 3 out]
                  n178 = Wait (ms)(milliseconds to wait=w340) -> ()  [unwired: 1 out]
                }
                frame #2 {
                  # "take N shots"
                  n179 = for {
                    N: 5 -> [_]
                    tunnel: w342 -> [w346]
                    tunnel: [w344] -> w341
                    n180 = Cancel Notification(0:w346) -> (8:w347:refnum<notifier>)  [unwired: 1 in, 2 out]
                    n181 = flat-sequence {
                      tunnel: w347 -> [w349]
                      tunnel: [w348] -> w345
                      tunnel: w345 -> [w359]
                      tunnel: [w358] -> w344
                      frame #0 {
                        n182 = while {
                          tunnel: w349 -> [w351]
                          tunnel: [w350] -> w348
                          stop <- w353 stop-if-true
                          # "wait for other loop\n to catch up"
                          # "wait till shooter is spun up and feeder is ready\nfor a short while"
                          n183 = local read "Shooter Happy"() -> (w356:bool)
                          n184 = local read "Feeder Happy"() -> (w355:bool)
                          n185 = Wait on Notification(notifier=w351, ignore previous (F)=FALSE) -> (notifier out=w350:refnum<notifier>)  [unwired: 2 in, 3 out]
                          n186 = And(x=w356, y=w355) -> (x .and. y?=w354:bool)
                          n187 = call "CheckShooter.vi"("Time for happy (ms)"=350.0, "Shooter Good?"=w354) -> ("Good to shoot"=w353:bool)  [unwired: 9 in]
                        }
                      }
                      frame #1 {
                        # "wait for other loop\n to catch up"
                        # "shoot the disk!!"
                        n188 = local write "Shoot!"(TRUE ("Shoot!")) -> ()
                        n189 = Wait on Notification(notifier=w359, ignore previous (F)=TRUE) -> (notifier out=w358:refnum<notifier>)  [unwired: 2 in, 3 out]
                      }
                    }
                  }
                }
                frame #3 {
                  # "wait for other loop\n to catch up"
                  # "wait for disk to\nexit shooter"
                  n190 = Wait on Notification(notifier=w362, ignore previous (F)=TRUE) -> (notifier out=w363:refnum<notifier>)  [unwired: 2 in, 3 out]
                  n191 = Wait (ms)(milliseconds to wait=u32 400) -> ()  [unwired: 1 out]
                }
                frame #4 {
                  # "wait for other loop\n to catch up"
                  # "set up for driving"
                  n192 = local write "Stop Drive"(FALSE ("Shift Low")) -> ()
                  n193 = local write "Shift Low"(TRUE ("Shift Low")) -> ()
                  n194 = Wait on Notification(notifier=w366, ignore previous (F)=TRUE) -> (notifier out=w367:refnum<notifier>)  [unwired: 2 in, 3 out]
                }
                frame #5 {
                  # "turn to faceaway\nfrom  goals\nstart at right side"
                  # "wait for other loop\n to catch up"
                  n195 = call "AutoTurnGyro.vi"("Turn Amount"=-30, "Initial Angle"=w373) -> ("Target Angle Out"=w371:dbl)  [unwired: 8 in, 1 out]
                  n196 = Wait on Notification(notifier=w374, ignore previous (F)=TRUE) -> (notifier out=w375:refnum<notifier>)  [unwired: 2 in, 3 out]
                }
                frame #6 {
                  # "wait for other loop\n to catch up"
                  # "drive backwars"
                  n197 = Wait on Notification(notifier=w382, ignore previous (F)=TRUE) -> (notifier out=w383:refnum<notifier>)  [unwired: 2 in, 3 out]
                  n198 = call "AutoDistanceGyro.vi"("InitialAngle"=w381, "Reset Encoders"=TRUE, "TargetDistance"=-54.0, "Motor Speed"=-0.6) -> ("InitialAngle Out"=w380:dbl)  [unwired: 10 in, 1 out]
                }
                frame #7 {
                  # "wait for other loop\n to catch up"
                  # "turn to face disks\nand start DAD and DT"
                  n199 = Wait on Notification(notifier=w388, ignore previous (F)=TRUE) -> (notifier out=w389:refnum<notifier>)  [unwired: 2 in, 3 out]
                  n200 = call "AutoTurnGyro.vi"("Turn Amount"=-90, "Initial Angle"=w386) -> ("Target Angle Out"=w385:dbl)  [unwired: 8 in, 1 out]
                }
                frame #8 {
                  # "wait for other loop\n to catch up"
                  # "start to drive over disks"
                  n201 = Wait on Notification(notifier=w399, ignore previous (F)=TRUE) -> (notifier out=w400:refnum<notifier>)  [unwired: 2 in, 3 out]
                  n202 = local write "DAD Output"(WPI_RelayValue."On" ("DAD Output")) -> ()
                  n203 = call "AutoDistanceGyro.vi"("InitialAngle"=w396, "Reset Encoders"=TRUE, "TargetDistance"=20.0, "Motor Speed"=0.6) -> ("InitialAngle Out"=w395:dbl)  [unwired: 10 in, 1 out]
                  n204 = local write "DT Output"(enum16{"Off", "Up", "Down"}."Up" ("DT Output")) -> ()
                  n205 = local write "DAD Up"(FALSE ("DAD Up")) -> ()
                }
                frame #9 {
                  # "after under pyramid\npop up shooter"
                  # "wait for other loop\n to catch up"
                  n206 = local write "Shooter Up"(TRUE ("DAD Up")) -> ()
                  n207 = Wait on Notification(notifier=w408, ignore previous (F)=TRUE) -> (notifier out=w407:refnum<notifier>)  [unwired: 2 in, 3 out]
                  n208 = call "AutoDistanceGyro.vi"("InitialAngle"=w404, "TargetDistance"=40.0, "Motor Speed"=0.6) -> ("InitialAngle Out"=w403:dbl)  [unwired: 11 in, 1 out]
                }
                frame #10 {
                  # "wait for pop up then\npop down"
                  # "wait for other loop\n to catch up"
                  n209 = local write "Shooter Up"(FALSE ("DAD Up")) -> ()
                  n210 = Wait on Notification(notifier=w415, ignore previous (F)=TRUE) -> (notifier out=w416:refnum<notifier>)  [unwired: 2 in, 3 out]
                  n211 = call "AutoDistanceGyro.vi"("InitialAngle"=w412, "TargetDistance"=112.0, "Motor Speed"=0.6) -> ("InitialAngle Out"=w411:dbl)  [unwired: 11 in, 1 out]
                }
                frame #11 {
                  # "wait for other loop\n to catch up"
                  # "turn to goals\nstart counting for\nDT slowness"
                  n212 = Wait on Notification(notifier=w422, ignore previous (F)=TRUE) -> (notifier out=w423:refnum<notifier>)  [unwired: 2 in, 3 out]
                  n213 = Tick Count (ms)() -> (millisecond timer value=w419:u32)
                  n214 = call "AutoTurnGyro.vi"("Turn Amount"=90, "Initial Angle"=w420) -> ("Target Angle Out"=w418:dbl)  [unwired: 8 in, 1 out]
                }
                frame #12 {
                  # "wait for other loop\n to catch up"
                  # "drive to close\npyramid"
                  n215 = Wait on Notification(notifier=w430, ignore previous (F)=TRUE) -> (notifier out=w431:refnum<notifier>)  [unwired: 2 in, 3 out]
                  n216 = call "AutoDistanceGyro.vi"("InitialAngle"=w427, "Reset Encoders"=TRUE, "TargetDistance"=54.0, "Motor Speed"=0.6) -> ("InitialAngle Out"=w425:dbl)  [unwired: 10 in, 1 out]
                }
                frame #13 {
                  # "aim at goals"
                  # "wait for other loop\n to catch up"
                  n217 = Wait on Notification(notifier=w436, ignore previous (F)=TRUE) -> (notifier out=w437:refnum<notifier>)  [unwired: 2 in, 3 out]
                  n218 = call "AutoTurnGyro.vi"("Turn Amount"=-60, "Initial Angle"=w434) -> ()  [unwired: 8 in, 2 out]
                }
                frame #14 {
                  # "wait for other loop\n to catch up"
                  # "make sure DT has caught up\nand finsih driving"
                  n219 = while {
                    tunnel: w441 -> [w447]
                    stop <- w450 stop-if-true
                    # "wait for 10 ms every\nloop not to hog resources"
                    n220 = Wait (ms)(milliseconds to wait=10) -> (millisecond timer value=w445:u32)
                    n221 = Add(x=w447, y=7000) -> (x+y=w446:u32)
                    n222 = Greater?(x=w445, y=w446) -> (0:w450:bool)
                  }
                  n223 = local write "Stop Drive"(TRUE ("Shift Low")) -> ()
                  n224 = Wait on Notification(notifier=w442, ignore previous (F)=TRUE) -> (notifier out=w443:refnum<notifier>)  [unwired: 2 in, 3 out]
                }
                frame #15 {
                  # "wait for other loop\n to catch up"
                  # "spend a split\nseccond turning\nstuff off"
                  n225 = local write "DAD Output"(WPI_RelayValue."Off" ("DAD Output")) -> ()
                  n226 = local write "DT Output"(enum16{"Off", "Up", "Down"}."Off" ("DT Output")) -> ()
                  n227 = local write "DAD Up"(TRUE ("DAD Up")) -> ()
                  n228 = Wait on Notification(notifier=w454, ignore previous (F)=TRUE) -> (notifier out=w455:refnum<notifier>)  [unwired: 2 in, 3 out]
                }
                frame #16 {
                  # "take N shots"
                  # "Shoot disks"
                  n229 = for {
                    N: 8 -> [_]
                    tunnel: w457 -> [w462]
                    tunnel: [w460] -> w458
                    n230 = Cancel Notification(0:w462) -> (8:w463:refnum<notifier>)  [unwired: 1 in, 2 out]
                    n231 = flat-sequence {
                      tunnel: w463 -> [w465]
                      tunnel: [w464] -> w461
                      tunnel: w461 -> [w475]
                      tunnel: [w474] -> w460
                      frame #0 {
                        n232 = while {
                          tunnel: w465 -> [w467]
                          tunnel: [w466] -> w464
                          stop <- w469 stop-if-true
                          # "wait for other loop\n to catch up"
                          # "wait till shooter is spun up and feeder is ready\nfor a short while"
                          n233 = local read "Shooter Happy"() -> (w472:bool)
                          n234 = local read "Feeder Happy"() -> (w471:bool)
                          n235 = Wait on Notification(notifier=w467, ignore previous (F)=FALSE) -> (notifier out=w466:refnum<notifier>)  [unwired: 2 in, 3 out]
                          n236 = And(x=w472, y=w471) -> (x .and. y?=w470:bool)
                          n237 = call "CheckShooter.vi"("Time for happy (ms)"=350.0, "Shooter Good?"=w470) -> ("Good to shoot"=w469:bool)  [unwired: 9 in]
                        }
                      }
                      frame #1 {
                        # "wait for other loop\n to catch up"
                        # "shoot the disk!!"
                        n238 = local write "Shoot!"(TRUE ("Shoot!")) -> ()
                        n239 = Wait on Notification(notifier=w475, ignore previous (F)=TRUE) -> (notifier out=w474:refnum<notifier>)  [unwired: 2 in, 3 out]
                      }
                    }
                  }
                }
                frame #17 {
                  # "make sure disks\nexist shooter"
                  # "wait for other loop\n to catch up"
                  n240 = Wait on Notification(notifier=w479, ignore previous (F)=TRUE) -> (notifier out=w480:refnum<notifier>)  [unwired: 2 in, 3 out]
                  n241 = Wait (ms)(milliseconds to wait=u32 750) -> ()  [unwired: 1 out]
                }
                frame #18 {
                  # "wait for other loop\n to catch up"
                  # "spin down shooter"
                  n242 = local write "Shooter Speed"(T3."Off" ("Shooter Speed")) -> ()
                  n243 = Wait on Notification(notifier=w483, ignore previous (F)=TRUE) -> (notifier out=w484:refnum<notifier>)  [unwired: 2 in, 3 out]
                }
                frame #19 {
                  # "wait for other loop\n to catch up"
                  # "finish auton mode"
                  n244 = local write "Auton Done"(TRUE ("Auton Done")) -> ()
                  n245 = Wait on Notification(notifier=w486, ignore previous (F)=TRUE) -> ()  [unwired: 2 in, 4 out]
                }
              }
            }
          }
        }
        frame 4 {
          n246 = case shown="1" w491 {
            tunnel: w490 -> [_ w502]
            tunnel: w489 -> [_ w497]
            frame 0, Default {
            }
            frame 1 {
              n247 = flat-sequence {
                tunnel: w502 -> [w506]
                tunnel: [w505] -> w499
                tunnel: w499 -> [w508]
                tunnel: [w509] -> w498
                tunnel: w497 -> [w512]
                tunnel: [w511] -> w496
                tunnel: w498 -> [w520]
                tunnel: [w516] -> w501
                tunnel: [w515] -> w500
                tunnel: w496 -> [w514]
                tunnel: w501 -> [w525]
                tunnel: w500 -> [w524]
                tunnel: [w523] -> w495
                tunnel: [w522] -> w492
                tunnel: w495 -> [w534]
                tunnel: [w530] -> w494
                tunnel: [w529] -> w493
                tunnel: w492 -> [w528]
                tunnel: w494 -> [w538]
                tunnel: w493 -> [w536]
                frame #0 {
                  # "wait for other loop\n to catch up"
                  n248 = local write "Stop Drive"(TRUE ("Stop Drive")) -> ()
                  n249 = local write "Shift Low"(TRUE ("Stop Drive")) -> ()
                  n250 = Wait on Notification(notifier=w506, ignore previous (F)=TRUE) -> (notifier out=w505:refnum<notifier>)  [unwired: 2 in, 3 out]
                }
                frame #1 {
                  # "wait for other loop\n to catch up"
                  n251 = call "AutoTurnGyro.vi"("Turn Amount"=-15, "Initial Angle"=w512) -> ("Target Angle Out"=w511:dbl)  [unwired: 8 in, 1 out]
                  n252 = Wait on Notification(notifier=w508, ignore previous (F)=TRUE) -> (notifier out=w509:refnum<notifier>)  [unwired: 2 in, 3 out]
                }
                frame #2 {
                  # "wait for other loop\n to catch up"
                  n253 = Wait on Notification(notifier=w520, ignore previous (F)=FALSE) -> (notifier out=w516:refnum<notifier>)  [unwired: 2 in, 3 out]
                  n254 = call "AutoDistanceGyro.vi"("InitialAngle"=w514, "Reset Encoders"=TRUE, "TargetDistance"=12 ("Turn Amount"), "Motor Speed"=1.0) -> ("InitialAngle Out"=w515:dbl)  [unwired: 10 in, 1 out]
                }
                frame #3 {
                  # "wait for other loop\n to catch up"
                  n255 = call "AutoTurnGyro.vi"("Turn Amount"=15, "Initial Angle"=w524) -> ("Target Angle Out"=w522:dbl)  [unwired: 8 in, 1 out]
                  n256 = Wait on Notification(notifier=w525, ignore previous (F)=TRUE) -> (notifier out=w523:refnum<notifier>)  [unwired: 2 in, 3 out]
                }
                frame #4 {
                  # "wait for other loop\n to catch up"
                  n257 = call "AutoDistanceGyro.vi"("InitialAngle"=w528, "Reset Encoders"=TRUE, "TargetDistance"=80 ("Turn Amount"), "Motor Speed"=1.0) -> ("InitialAngle Out"=w529:dbl)  [unwired: 10 in, 1 out]
                  n258 = Wait on Notification(notifier=w534, ignore previous (F)=TRUE) -> (notifier out=w530:refnum<notifier>)  [unwired: 2 in, 3 out]
                }
                frame #5 {
                  # "wait for other loop\n to catch up"
                  n259 = call "AutoTurnGyro.vi"("Turn Amount"=-30, "Initial Angle"=w536) -> ()  [unwired: 8 in, 2 out]
                  n260 = Wait on Notification(notifier=w538, ignore previous (F)=TRUE) -> ()  [unwired: 2 in, 4 out]
                }
              }
            }
          }
        }
        frame 5 {
          n261 = case shown="2" w543 {
            tunnel: w542 -> [_ w551 w632]
            tunnel: w541 -> [_ w554 w635]
            tunnel: w540 -> [_ w544 w625]
            frame 0, Default {
              # "do nothing"
            }
            frame 1 {
              # "2 shots, back of pyramid --> done"
              n262 = flat-sequence {
                tunnel: [w558] -> w553
                tunnel: w551 -> [w557]
                tunnel: w554 -> [w563]
                tunnel: w553 -> [w561]
                tunnel: [w560] -> w552
                tunnel: w552 -> [w567]
                tunnel: [w566] -> w549
                tunnel: [w602] -> w550
                tunnel: w549 -> [w601]
                tunnel: [w607] -> w548
                tunnel: w550 -> [w606]
                tunnel: w548 -> [w611]
                tunnel: [w612] -> w545
                tunnel: w544 -> [w609]
                tunnel: [w615] -> w546
                tunnel: w545 -> [w614]
                tunnel: [w618] -> w547
                tunnel: w546 -> [w617]
                tunnel: w547 -> [w620]
                frame #0 {
                  # "wait for other loop\n to catch up"
                  # "spin up shooter"
                  n263 = local write "Shoot!"(FALSE ("Shoot!")) -> ()
                  n264 = local write "Shooter Speed"(T1."Far Pyramid 3pt" ("Shooter Speed")) -> ()
                  n265 = Wait on Notification(notifier=w557, ignore previous (F)=TRUE) -> (notifier out=w558:refnum<notifier>)  [unwired: 2 in, 3 out]
                }
                frame #1 {
                  # "wait for other loop\n to catch up"
                  # "wait [delay] * 1000 ms\nwhich is [delay] seconds"
                  n266 = Multiply(x=w563, y=1000) -> (x*y=w565:u32)
                  n267 = Wait on Notification(notifier=w561, ignore previous (F)=FALSE) -> (notifier out=w560:refnum<notifier>)  [unwired: 2 in, 3 out]
                  n268 = Wait (ms)(milliseconds to wait=w565) -> ()  [unwired: 1 out]
                }
                frame #2 {
                  # "take N shots"
                  n269 = for {
                    N: 2 -> [_]
                    tunnel: w567 -> [w573]
                    tunnel: [w571] -> w566
                    n270 = Cancel Notification(0:w573) -> (8:w574:refnum<notifier>)  [unwired: 1 in, 2 out]
                    n271 = flat-sequence {
                      tunnel: w574 -> [w576]
                      tunnel: [w575] -> w572
                      tunnel: w572 -> [w586]
                      tunnel: [w585] -> w570
                      tunnel: w570 -> [w589]
                      tunnel: [w590] -> w569
                      tunnel: [w599] -> w571
                      tunnel: w569 -> [w598]
                      frame #0 {
                        n272 = while {
                          tunnel: w576 -> [w578]
                          tunnel: [w577] -> w575
                          stop <- w580 stop-if-true
                          # "if spin up for too long\ndisk might not slow\nshooter down enough"
                          # "wait for other loop\n to catch up"
                          # "wait till shooter is spun up and feeder is ready\nfor a short while"
                          n273 = local read "Shooter Happy"() -> (w583:bool)
                          n274 = local read "Feeder Happy"() -> (w582:bool)
                          n275 = Wait on Notification(notifier=w578, ignore previous (F)=FALSE) -> (notifier out=w577:refnum<notifier>)  [unwired: 2 in, 3 out]
                          n276 = And(x=w583, y=w582) -> (x .and. y?=w581:bool)
                          n277 = call "CheckShooter.vi"("Time for happy (ms)"=50.0, "Shooter Good?"=w581) -> ("Good to shoot"=w580:bool)  [unwired: 9 in]
                        }
                      }
                      frame #1 {
                        # "wait for other loop\n to catch up"
                        # "shoot the disk!!"
                        n278 = local write "Shoot!"(TRUE ("Shoot!")) -> ()
                        n279 = Wait on Notification(notifier=w586, ignore previous (F)=TRUE) -> (notifier out=w585:refnum<notifier>)  [unwired: 2 in, 3 out]
                      }
                      frame #2 {
                        n280 = disable-structure shown="Enabled" {
                          disable-tunnel: [w592 _] -> w590
                          disable-tunnel: w589 -> [w591 _]
                          frame Enabled {
                            # "wait for other loop\n to catch up"
                            n281 = while {
                              stop <- w596 stop-if-true
                              # "wait for shooter to slow\ndown bc disk exited"
                              n282 = local read "Shooter Happy"() -> (w595:bool)
                              n283 = Wait (ms)(milliseconds to wait=u32 10) -> ()  [unwired: 1 out]
                              n284 = Not(x=w595) -> (.not. x?=w596:bool)
                            }
                            n285 = Wait on Notification(notifier=w591, ignore previous (F)=FALSE) -> (notifier out=w592:refnum<notifier>)  [unwired: 2 in, 3 out]
                          }
                          frame Disabled {
                          }
                        }
                      }
                      frame #3 {
                        # "once disk has exited\nstop trying to shoot"
                        # "wait for other loop\n to catch up"
                        n286 = local write "Shoot!"(FALSE) -> ()
                        n287 = Wait on Notification(notifier=w598, ignore previous (F)=TRUE) -> (notifier out=w599:refnum<notifier>)  [unwired: 2 in, 3 out]
                      }
                    }
                  }
                }
                frame #3 {
                  # "wait for other loop\n to catch up"
                  # "wait for disk to\nexit shooter"
                  n288 = Wait on Notification(notifier=w601, ignore previous (F)=TRUE) -> (notifier out=w602:refnum<notifier>)  [unwired: 2 in, 3 out]
                  n289 = Wait (ms)(milliseconds to wait=u32 500) -> ()  [unwired: 1 out]
                }
                frame #4 {
                  # "wait for other loop\n to catch up"
                  # "spin down shooter"
                  n290 = local write "Shooter Speed"(T3."Off" ("Shooter Speed")) -> ()
                  n291 = Wait on Notification(notifier=w606, ignore previous (F)=TRUE) -> (notifier out=w607:refnum<notifier>)  [unwired: 2 in, 3 out]
                }
                frame #5 {
                  # "wait for other loop\n to catch up"
                  n292 = Wait on Notification(notifier=w611, ignore previous (F)=FALSE) -> (notifier out=w612:refnum<notifier>)  [unwired: 2 in, 3 out]
                  n293 = call "AutoTurnGyro.vi"("Turn Amount"=-30, "Initial Angle"=w609) -> ()  [unwired: 8 in, 2 out]
                }
                frame #6 {
                  # "wait for other loop\n to catch up"
                  n294 = Wait on Notification(notifier=w614, ignore previous (F)=TRUE) -> (notifier out=w615:refnum<notifier>)  [unwired: 2 in, 3 out]
                }
                frame #7 {
                  # "wait for other loop\n to catch up"
                  n295 = Wait on Notification(notifier=w617, ignore previous (F)=TRUE) -> (notifier out=w618:refnum<notifier>)  [unwired: 2 in, 3 out]
                }
                frame #8 {
                  # "wait for other loop\n to catch up"
                  # "finish auton mode"
                  n296 = local write "Auton Done"(TRUE ("Auton Done")) -> ()
                  n297 = Wait on Notification(notifier=w620, ignore previous (F)=FALSE) -> ()  [unwired: 2 in, 4 out]
                }
              }
            }
            frame 2 {
              # "3 shots, back of pyramid --> done"
              n298 = flat-sequence {
                tunnel: [w639] -> w634
                tunnel: w632 -> [w638]
                tunnel: w635 -> [w644]
                tunnel: w634 -> [w642]
                tunnel: [w641] -> w633
                tunnel: w633 -> [w648]
                tunnel: [w647] -> w630
                tunnel: [w683] -> w631
                tunnel: w630 -> [w682]
                tunnel: [w688] -> w629
                tunnel: w631 -> [w687]
                tunnel: w629 -> [w696]
                tunnel: [w697] -> w626
                tunnel: w625 -> [w691]
                tunnel: [w692] -> w624
                tunnel: [w705] -> w627
                tunnel: w626 -> [w704]
                tunnel: w624 -> [w702]
                tunnel: [w701] -> w623
                tunnel: [w714] -> w628
                tunnel: w627 -> [w713]
                tunnel: w623 -> [w709]
                tunnel: w628 -> [w716]
                frame #0 {
                  # "wait for other loop\n to catch up"
                  # "spin up shooter"
                  n299 = local write "Shoot!"(FALSE ("Shoot!")) -> ()
                  n300 = local write "Shooter Speed"(T1."Far Pyramid 3pt" ("Shooter Speed")) -> ()
                  n301 = Wait on Notification(notifier=w638, ignore previous (F)=TRUE) -> (notifier out=w639:refnum<notifier>)  [unwired: 2 in, 3 out]
                }
                frame #1 {
                  # "wait for other loop\n to catch up"
                  # "wait [delay] * 1000 ms\nwhich is [delay] seconds"
                  n302 = Multiply(x=w644, y=1000) -> (x*y=w646:u32)
                  n303 = Wait on Notification(notifier=w642, ignore previous (F)=FALSE) -> (notifier out=w641:refnum<notifier>)  [unwired: 2 in, 3 out]
                  n304 = Wait (ms)(milliseconds to wait=w646) -> ()  [unwired: 1 out]
                }
                frame #2 {
                  # "take N shots"
                  n305 = for {
                    N: 3 -> [_]
                    tunnel: w648 -> [w654]
                    tunnel: [w652] -> w647
                    n306 = Cancel Notification(0:w654) -> (8:w655:refnum<notifier>)  [unwired: 1 in, 2 out]
                    n307 = flat-sequence {
                      tunnel: w655 -> [w657]
                      tunnel: [w656] -> w653
                      tunnel: w653 -> [w667]
                      tunnel: [w666] -> w651
                      tunnel: w651 -> [w670]
                      tunnel: [w671] -> w650
                      tunnel: [w680] -> w652
                      tunnel: w650 -> [w679]
                      frame #0 {
                        n308 = while {
                          tunnel: w657 -> [w659]
                          tunnel: [w658] -> w656
                          stop <- w661 stop-if-true
                          # "if spin up for too long\ndisk might not slow\nshooter down enough"
                          # "wait for other loop\n to catch up"
                          # "wait till shooter is spun up and feeder is ready\nfor a short while"
                          n309 = local read "Shooter Happy"() -> (w664:bool)
                          n310 = local read "Feeder Happy"() -> (w663:bool)
                          n311 = Wait on Notification(notifier=w659, ignore previous (F)=FALSE) -> (notifier out=w658:refnum<notifier>)  [unwired: 2 in, 3 out]
                          n312 = And(x=w664, y=w663) -> (x .and. y?=w662:bool)
                          n313 = call "CheckShooter.vi"("Time for happy (ms)"=50.0, "Shooter Good?"=w662) -> ("Good to shoot"=w661:bool)  [unwired: 9 in]
                        }
                      }
                      frame #1 {
                        # "wait for other loop\n to catch up"
                        # "shoot the disk!!"
                        n314 = local write "Shoot!"(TRUE ("Shoot!")) -> ()
                        n315 = Wait on Notification(notifier=w667, ignore previous (F)=TRUE) -> (notifier out=w666:refnum<notifier>)  [unwired: 2 in, 3 out]
                      }
                      frame #2 {
                        n316 = disable-structure shown="Enabled" {
                          disable-tunnel: [w673 _] -> w671
                          disable-tunnel: w670 -> [w672 _]
                          frame Enabled {
                            # "wait for other loop\n to catch up"
                            n317 = while {
                              stop <- w677 stop-if-true
                              # "wait for shooter to slow\ndown bc disk exited"
                              n318 = local read "Shooter Happy"() -> (w676:bool)
                              n319 = Wait (ms)(milliseconds to wait=u32 10) -> ()  [unwired: 1 out]
                              n320 = Not(x=w676) -> (.not. x?=w677:bool)
                            }
                            n321 = Wait on Notification(notifier=w672, ignore previous (F)=FALSE) -> (notifier out=w673:refnum<notifier>)  [unwired: 2 in, 3 out]
                          }
                          frame Disabled {
                          }
                        }
                      }
                      frame #3 {
                        # "once disk has exited\nstop trying to shoot"
                        # "wait for other loop\n to catch up"
                        n322 = local write "Shoot!"(FALSE) -> ()
                        n323 = Wait on Notification(notifier=w679, ignore previous (F)=TRUE) -> (notifier out=w680:refnum<notifier>)  [unwired: 2 in, 3 out]
                      }
                    }
                  }
                }
                frame #3 {
                  # "wait for other loop\n to catch up"
                  # "wait for disk to\nexit shooter"
                  n324 = Wait on Notification(notifier=w682, ignore previous (F)=TRUE) -> (notifier out=w683:refnum<notifier>)  [unwired: 2 in, 3 out]
                  n325 = Wait (ms)(milliseconds to wait=u32 500) -> ()  [unwired: 1 out]
                }
                frame #4 {
                  # "wait for other loop\n to catch up"
                  # "spin down shooter"
                  n326 = local write "Shooter Speed"(T3."Off" ("Shooter Speed")) -> ()
                  n327 = Wait on Notification(notifier=w687, ignore previous (F)=TRUE) -> (notifier out=w688:refnum<notifier>)  [unwired: 2 in, 3 out]
                }
                frame #5 {
                  # "back off pyramid"
                  # "wait for other loop\n to catch up"
                  n328 = Wait on Notification(notifier=w696, ignore previous (F)=FALSE) -> (notifier out=w697:refnum<notifier>)  [unwired: 2 in, 3 out]
                  n329 = call "AutoDistanceGyro.vi"("InitialAngle"=w691, "Reset Encoders"=TRUE, "Sensor (Gyro)"=enum16{"Gyro", "Encoder"}."Encoder", "TargetDistance"=-12.0, "Motor Speed"=-0.6) -> ("InitialAngle Out"=w692:dbl)  [unwired: 9 in, 1 out]
                }
                frame #6 {
                  # "on left side\nturn CW"
                  # "wait for other loop\n to catch up"
                  n330 = local write "Shooter Up"(TRUE ("Shooter Up")) -> ()
                  n331 = Wait on Notification(notifier=w704, ignore previous (F)=TRUE) -> (notifier out=w705:refnum<notifier>)  [unwired: 2 in, 3 out]
                  n332 = call "AutoTurnGyro.vi"("Sensor (Gyro)"=enum16{"Gyro", "Vision", "Encoder"}."Encoder", "Turn Amount"=-70, "Initial Angle"=w702) -> ("Target Angle Out"=w701:dbl)  [unwired: 7 in, 1 out]
                }
                frame #7 {
                  # "back towards \ncenterline"
                  # "wait for other loop\n to catch up"
                  n333 = local write "Shooter Up"(FALSE ("Shooter Up")) -> ()
                  n334 = Wait on Notification(notifier=w713, ignore previous (F)=TRUE) -> (notifier out=w714:refnum<notifier>)  [unwired: 2 in, 3 out]
                  n335 = call "AutoDistanceGyro.vi"("InitialAngle"=w709, "Reset Encoders"=TRUE, "Sensor (Gyro)"=enum16{"Gyro", "Encoder"}."Encoder", "TargetDistance"=-36.0, "Motor Speed"=-1.0) -> ()  [unwired: 9 in, 2 out]
                }
                frame #8 {
                  # "wait for other loop\n to catch up"
                  # "finish auton mode"
                  n336 = local write "Auton Done"(TRUE ("Auton Done")) -> ()
                  n337 = Wait on Notification(notifier=w716, ignore previous (F)=FALSE) -> ()  [unwired: 2 in, 4 out]
                }
              }
            }
          }
        }
        frame 6 {
          n338 = case shown="2" w722 {
            tunnel: w721 -> [_ w730 w811]
            tunnel: w720 -> [_ w733 w814]
            tunnel: w719 -> [_ w723 w804]
            frame 0, Default {
              # "do nothing"
            }
            frame 1 {
              # "2 shots, back of pyramid --> done"
              n339 = flat-sequence {
                tunnel: [w737] -> w732
                tunnel: w730 -> [w736]
                tunnel: w733 -> [w742]
                tunnel: w732 -> [w740]
                tunnel: [w739] -> w731
                tunnel: w731 -> [w746]
                tunnel: [w745] -> w728
                tunnel: [w781] -> w729
                tunnel: w728 -> [w780]
                tunnel: [w786] -> w727
                tunnel: w729 -> [w785]
                tunnel: w727 -> [w790]
                tunnel: [w791] -> w724
                tunnel: w723 -> [w788]
                tunnel: [w794] -> w725
                tunnel: w724 -> [w793]
                tunnel: [w797] -> w726
                tunnel: w725 -> [w796]
                tunnel: w726 -> [w799]
                frame #0 {
                  # "wait for other loop\n to catch up"
                  # "spin up shooter"
                  n340 = local write "Shoot!"(FALSE ("Shoot!")) -> ()
                  n341 = local write "Shooter Speed"(T1."Far Pyramid 3pt" ("Shooter Speed")) -> ()
                  n342 = Wait on Notification(notifier=w736, ignore previous (F)=TRUE) -> (notifier out=w737:refnum<notifier>)  [unwired: 2 in, 3 out]
                }
                frame #1 {
                  # "wait for other loop\n to catch up"
                  # "wait [delay] * 1000 ms\nwhich is [delay] seconds"
                  n343 = Multiply(x=w742, y=1000) -> (x*y=w744:u32)
                  n344 = Wait on Notification(notifier=w740, ignore previous (F)=FALSE) -> (notifier out=w739:refnum<notifier>)  [unwired: 2 in, 3 out]
                  n345 = Wait (ms)(milliseconds to wait=w744) -> ()  [unwired: 1 out]
                }
                frame #2 {
                  # "take N shots"
                  n346 = for {
                    N: 2 -> [_]
                    tunnel: w746 -> [w752]
                    tunnel: [w750] -> w745
                    n347 = Cancel Notification(0:w752) -> (8:w753:refnum<notifier>)  [unwired: 1 in, 2 out]
                    n348 = flat-sequence {
                      tunnel: w753 -> [w755]
                      tunnel: [w754] -> w751
                      tunnel: w751 -> [w765]
                      tunnel: [w764] -> w749
                      tunnel: w749 -> [w768]
                      tunnel: [w769] -> w748
                      tunnel: [w778] -> w750
                      tunnel: w748 -> [w777]
                      frame #0 {
                        n349 = while {
                          tunnel: w755 -> [w757]
                          tunnel: [w756] -> w754
                          stop <- w759 stop-if-true
                          # "if spin up for too long\ndisk might not slow\nshooter down enough"
                          # "wait for other loop\n to catch up"
                          # "wait till shooter is spun up and feeder is ready\nfor a short while"
                          n350 = local read "Shooter Happy"() -> (w762:bool)
                          n351 = local read "Feeder Happy"() -> (w761:bool)
                          n352 = Wait on Notification(notifier=w757, ignore previous (F)=FALSE) -> (notifier out=w756:refnum<notifier>)  [unwired: 2 in, 3 out]
                          n353 = And(x=w762, y=w761) -> (x .and. y?=w760:bool)
                          n354 = call "CheckShooter.vi"("Time for happy (ms)"=50.0, "Shooter Good?"=w760) -> ("Good to shoot"=w759:bool)  [unwired: 9 in]
                        }
                      }
                      frame #1 {
                        # "wait for other loop\n to catch up"
                        # "shoot the disk!!"
                        n355 = local write "Shoot!"(TRUE ("Shoot!")) -> ()
                        n356 = Wait on Notification(notifier=w765, ignore previous (F)=TRUE) -> (notifier out=w764:refnum<notifier>)  [unwired: 2 in, 3 out]
                      }
                      frame #2 {
                        n357 = disable-structure shown="Enabled" {
                          disable-tunnel: [w771 _] -> w769
                          disable-tunnel: w768 -> [w770 _]
                          frame Enabled {
                            # "wait for other loop\n to catch up"
                            n358 = while {
                              stop <- w775 stop-if-true
                              # "wait for shooter to slow\ndown bc disk exited"
                              n359 = local read "Shooter Happy"() -> (w774:bool)
                              n360 = Wait (ms)(milliseconds to wait=u32 10) -> ()  [unwired: 1 out]
                              n361 = Not(x=w774) -> (.not. x?=w775:bool)
                            }
                            n362 = Wait on Notification(notifier=w770, ignore previous (F)=FALSE) -> (notifier out=w771:refnum<notifier>)  [unwired: 2 in, 3 out]
                          }
                          frame Disabled {
                          }
                        }
                      }
                      frame #3 {
                        # "once disk has exited\nstop trying to shoot"
                        # "wait for other loop\n to catch up"
                        n363 = local write "Shoot!"(FALSE) -> ()
                        n364 = Wait on Notification(notifier=w777, ignore previous (F)=TRUE) -> (notifier out=w778:refnum<notifier>)  [unwired: 2 in, 3 out]
                      }
                    }
                  }
                }
                frame #3 {
                  # "wait for other loop\n to catch up"
                  # "wait for disk to\nexit shooter"
                  n365 = Wait on Notification(notifier=w780, ignore previous (F)=TRUE) -> (notifier out=w781:refnum<notifier>)  [unwired: 2 in, 3 out]
                  n366 = Wait (ms)(milliseconds to wait=u32 500) -> ()  [unwired: 1 out]
                }
                frame #4 {
                  # "wait for other loop\n to catch up"
                  # "spin down shooter"
                  n367 = local write "Shooter Speed"(T3."Off" ("Shooter Speed")) -> ()
                  n368 = Wait on Notification(notifier=w785, ignore previous (F)=TRUE) -> (notifier out=w786:refnum<notifier>)  [unwired: 2 in, 3 out]
                }
                frame #5 {
                  # "wait for other loop\n to catch up"
                  n369 = Wait on Notification(notifier=w790, ignore previous (F)=FALSE) -> (notifier out=w791:refnum<notifier>)  [unwired: 2 in, 3 out]
                  n370 = call "AutoTurnGyro.vi"("Turn Amount"=-30, "Initial Angle"=w788) -> ()  [unwired: 8 in, 2 out]
                }
                frame #6 {
                  # "wait for other loop\n to catch up"
                  n371 = Wait on Notification(notifier=w793, ignore previous (F)=TRUE) -> (notifier out=w794:refnum<notifier>)  [unwired: 2 in, 3 out]
                }
                frame #7 {
                  # "wait for other loop\n to catch up"
                  n372 = Wait on Notification(notifier=w796, ignore previous (F)=TRUE) -> (notifier out=w797:refnum<notifier>)  [unwired: 2 in, 3 out]
                }
                frame #8 {
                  # "wait for other loop\n to catch up"
                  # "finish auton mode"
                  n373 = local write "Auton Done"(TRUE ("Auton Done")) -> ()
                  n374 = Wait on Notification(notifier=w799, ignore previous (F)=FALSE) -> ()  [unwired: 2 in, 4 out]
                }
              }
            }
            frame 2 {
              # "3 shots, back of pyramid --> done"
              n375 = flat-sequence {
                tunnel: [w818] -> w813
                tunnel: w811 -> [w817]
                tunnel: w814 -> [w823]
                tunnel: w813 -> [w821]
                tunnel: [w820] -> w812
                tunnel: w812 -> [w827]
                tunnel: [w826] -> w809
                tunnel: [w864] -> w810
                tunnel: w809 -> [w863]
                tunnel: [w869] -> w808
                tunnel: w810 -> [w868]
                tunnel: w808 -> [w877]
                tunnel: [w878] -> w805
                tunnel: w804 -> [w872]
                tunnel: [w873] -> w803
                tunnel: [w886] -> w806
                tunnel: w805 -> [w885]
                tunnel: w803 -> [w883]
                tunnel: [w882] -> w802
                tunnel: [w895] -> w807
                tunnel: w806 -> [w894]
                tunnel: w802 -> [w890]
                tunnel: w807 -> [w897]
                frame #0 {
                  # "wait for other loop\n to catch up"
                  # "spin up shooter"
                  n376 = local write "Shoot!"(FALSE ("Shoot!")) -> ()
                  n377 = local write "Shooter Speed"(T1."Far Pyramid 3pt" ("Shooter Speed")) -> ()
                  n378 = Wait on Notification(notifier=w817, ignore previous (F)=TRUE) -> (notifier out=w818:refnum<notifier>)  [unwired: 2 in, 3 out]
                }
                frame #1 {
                  # "wait for other loop\n to catch up"
                  # "wait [delay] * 1000 ms\nwhich is [delay] seconds"
                  n379 = Multiply(x=w823, y=1000) -> (x*y=w825:u32)
                  n380 = Wait on Notification(notifier=w821, ignore previous (F)=FALSE) -> (notifier out=w820:refnum<notifier>)  [unwired: 2 in, 3 out]
                  n381 = Wait (ms)(milliseconds to wait=w825) -> ()  [unwired: 1 out]
                }
                frame #2 {
                  n382 = disable-structure shown="Enabled" {
                    disable-tunnel: w827 -> [w829 _]
                    disable-tunnel: [w828 _] -> w826
                    frame Disabled {
                      # "take N shots"
                      n383 = for {
                        N: 3 -> [_]
                        tunnel: w829 -> [w835]
                        tunnel: [w833] -> w828
                        n384 = Cancel Notification(0:w835) -> (8:w836:refnum<notifier>)  [unwired: 1 in, 2 out]
                        n385 = flat-sequence {
                          tunnel: w836 -> [w838]
                          tunnel: [w837] -> w834
                          tunnel: w834 -> [w848]
                          tunnel: [w847] -> w832
                          tunnel: w832 -> [w851]
                          tunnel: [w852] -> w831
                          tunnel: [w861] -> w833
                          tunnel: w831 -> [w860]
                          frame #0 {
                            n386 = while {
                              tunnel: w838 -> [w840]
                              tunnel: [w839] -> w837
                              stop <- w842 stop-if-true
                              # "if spin up for too long\ndisk might not slow\nshooter down enough"
                              # "wait for other loop\n to catch up"
                              # "wait till shooter is spun up and feeder is ready\nfor a short while"
                              n387 = local read "Shooter Happy"() -> (w845:bool)
                              n388 = local read "Feeder Happy"() -> (w844:bool)
                              n389 = Wait on Notification(notifier=w840, ignore previous (F)=FALSE) -> (notifier out=w839:refnum<notifier>)  [unwired: 2 in, 3 out]
                              n390 = And(x=w845, y=w844) -> (x .and. y?=w843:bool)
                              n391 = call "CheckShooter.vi"("Time for happy (ms)"=50.0, "Shooter Good?"=w843) -> ("Good to shoot"=w842:bool)  [unwired: 9 in]
                            }
                          }
                          frame #1 {
                            # "wait for other loop\n to catch up"
                            # "shoot the disk!!"
                            n392 = local write "Shoot!"(TRUE ("Shoot!")) -> ()
                            n393 = Wait on Notification(notifier=w848, ignore previous (F)=TRUE) -> (notifier out=w847:refnum<notifier>)  [unwired: 2 in, 3 out]
                          }
                          frame #2 {
                            n394 = disable-structure shown="Enabled" {
                              disable-tunnel: [w854 _] -> w852
                              disable-tunnel: w851 -> [w853 _]
                              frame Enabled {
                                # "wait for other loop\n to catch up"
                                n395 = while {
                                stop <- w858 stop-if-true
                                # "wait for shooter to slow\ndown bc disk exited"
                                n396 = local read "Shooter Happy"() -> (w857:bool)
                                n397 = Wait (ms)(milliseconds to wait=u32 10) -> ()  [unwired: 1 out]
                                n398 = Not(x=w857) -> (.not. x?=w858:bool)
                                }
                                n399 = Wait on Notification(notifier=w853, ignore previous (F)=FALSE) -> (notifier out=w854:refnum<notifier>)  [unwired: 2 in, 3 out]
                              }
                              frame Disabled {
                              }
                            }
                          }
                          frame #3 {
                            # "once disk has exited\nstop trying to shoot"
                            # "wait for other loop\n to catch up"
                            n400 = local write "Shoot!"(FALSE) -> ()
                            n401 = Wait on Notification(notifier=w860, ignore previous (F)=TRUE) -> (notifier out=w861:refnum<notifier>)  [unwired: 2 in, 3 out]
                          }
                        }
                      }
                    }
                    frame Enabled {
                    }
                  }
                }
                frame #3 {
                  # "wait for other loop\n to catch up"
                  # "wait for disk to\nexit shooter"
                  n402 = Wait on Notification(notifier=w863, ignore previous (F)=TRUE) -> (notifier out=w864:refnum<notifier>)  [unwired: 2 in, 3 out]
                  n403 = Wait (ms)(milliseconds to wait=u32 500) -> ()  [unwired: 1 out]
                }
                frame #4 {
                  # "wait for other loop\n to catch up"
                  # "spin down shooter"
                  n404 = local write "Shooter Speed"(T3."Off" ("Shooter Speed")) -> ()
                  n405 = Wait on Notification(notifier=w868, ignore previous (F)=TRUE) -> (notifier out=w869:refnum<notifier>)  [unwired: 2 in, 3 out]
                }
                frame #5 {
                  # "back off pyramid"
                  # "wait for other loop\n to catch up"
                  n406 = Wait on Notification(notifier=w877, ignore previous (F)=FALSE) -> (notifier out=w878:refnum<notifier>)  [unwired: 2 in, 3 out]
                  n407 = call "AutoDistanceGyro.vi"("InitialAngle"=w872, "Reset Encoders"=TRUE, "Sensor (Gyro)"=enum16{"Gyro", "Encoder"}."Encoder", "TargetDistance"=-12.0, "Motor Speed"=-0.6) -> ("InitialAngle Out"=w873:dbl)  [unwired: 9 in, 1 out]
                }
                frame #6 {
                  # "on right side\nturn a lot CW"
                  # "wait for other loop\n to catch up"
                  n408 = local write "Shooter Up"(TRUE ("Shooter Up")) -> ()
                  n409 = Wait on Notification(notifier=w885, ignore previous (F)=TRUE) -> (notifier out=w886:refnum<notifier>)  [unwired: 2 in, 3 out]
                  n410 = call "AutoTurnGyro.vi"("Sensor (Gyro)"=enum16{"Gyro", "Vision", "Encoder"}."Encoder", "Turn Amount"=-120, "Initial Angle"=w883) -> ("Target Angle Out"=w882:dbl)  [unwired: 7 in, 1 out]
                }
                frame #7 {
                  # "back towards \ncenterline"
                  # "wait for other loop\n to catch up"
                  n411 = local write "Shooter Up"(FALSE ("Shooter Up")) -> ()
                  n412 = Wait on Notification(notifier=w894, ignore previous (F)=TRUE) -> (notifier out=w895:refnum<notifier>)  [unwired: 2 in, 3 out]
                  n413 = call "AutoDistanceGyro.vi"("InitialAngle"=w890, "Reset Encoders"=TRUE, "Sensor (Gyro)"=enum16{"Gyro", "Encoder"}."Encoder", "TargetDistance"=-36.0, "Motor Speed"=-1.0) -> ()  [unwired: 9 in, 2 out]
                }
                frame #8 {
                  # "wait for other loop\n to catch up"
                  # "finish auton mode"
                  n414 = local write "Auton Done"(TRUE ("Auton Done")) -> ()
                  n415 = Wait on Notification(notifier=w897, ignore previous (F)=FALSE) -> ()  [unwired: 2 in, 4 out]
                }
              }
            }
          }
        }
        frame 9 {
          n416 = case shown="2" w902 {
            tunnel: w901 -> [_ w904 w914 w926]
            tunnel: w900 -> [_ _ w912 w924]
            frame 0, Default {
            }
            frame 1 {
              n417 = flat-sequence {
                tunnel: w904 -> [w908]
                tunnel: [w907] -> w903
                tunnel: w903 -> [w910]
                frame #0 {
                  # "wait for other loop\n to catch up"
                  n418 = local write "Stop Drive"(TRUE ("Stop Drive")) -> ()
                  n419 = local write "Shift Low"(TRUE ("Stop Drive")) -> ()
                  n420 = Wait on Notification(notifier=w908, ignore previous (F)=TRUE) -> (notifier out=w907:refnum<notifier>)  [unwired: 2 in, 3 out]
                }
                frame #1 {
                  # "wait for other loop\n to catch up"
                  n421 = call "Manual Turn.vi"() -> ()  [unwired: 12 in]
                  n422 = Wait on Notification(notifier=w910, ignore previous (F)=FALSE) -> ()  [unwired: 2 in, 4 out]
                }
              }
            }
            frame 2 {
              n423 = flat-sequence {
                tunnel: w914 -> [w918]
                tunnel: [w917] -> w913
                tunnel: w913 -> [w922]
                tunnel: w912 -> [_]
                frame #0 {
                  # "wait for other loop\n to catch up"
                  n424 = local write "Stop Drive"(TRUE ("Stop Drive")) -> ()
                  n425 = local write "Shift Low"(TRUE ("Stop Drive")) -> ()
                  n426 = Wait on Notification(notifier=w918, ignore previous (F)=TRUE) -> (notifier out=w917:refnum<notifier>)  [unwired: 2 in, 3 out]
                }
                frame #1 {
                  # "wait for other loop\n to catch up"
                  n427 = call "AutoTurnGyro.vi"("Turn Amount"=-15, "Initial Angle"=0.0) -> ()  [unwired: 8 in, 2 out]
                  n428 = Wait on Notification(notifier=w922, ignore previous (F)=FALSE) -> ()  [unwired: 2 in, 4 out]
                }
              }
            }
            frame 3 {
              n429 = flat-sequence {
                tunnel: w926 -> [w930]
                tunnel: [w929] -> w925
                tunnel: w925 -> [w936]
                tunnel: w924 -> [_]
                frame #0 {
                  # "wait for other loop\n to catch up"
                  n430 = local write "Stop Drive"(TRUE ("Stop Drive")) -> ()
                  n431 = local write "Shift Low"(TRUE ("Stop Drive")) -> ()
                  n432 = Wait on Notification(notifier=w930, ignore previous (F)=TRUE) -> (notifier out=w929:refnum<notifier>)  [unwired: 2 in, 3 out]
                }
                frame #1 {
                  # "wait for other loop\n to catch up"
                  n433 = Wait on Notification(notifier=w936, ignore previous (F)=FALSE) -> ()  [unwired: 2 in, 4 out]
                  n434 = call "AutoDistanceGyro.vi"("InitialAngle"=0.0 ("Initial Angle"), "Reset Encoders"=TRUE, "TargetDistance"=102 ("Turn Amount"), "Motor Speed"=1.0) -> ()  [unwired: 10 in, 2 out]
                }
              }
            }
          }
        }
      }
    }
  }
